vi "Preset_Manager_Main_Integrated.vi"(0 "Cluster":cluster{"Numeric":dbl}, 1 "All Devices Core Info":string[][](array[string]), 2 "Virtual Devices List":string[](array[string]), 3 "Filtered Devices List":string[](array[string]), 4 "DevStatusQueue":refnum<queue>, 5 "UDP timeout ms":i32, 6 "MC Multicast":refnum<k16>, 7 "MCast Remote":u16, 8 "My IP":string, 9 "Experiment Name":string, 10 "Software Root":string, 11 "Mcast address":string) -> ()   [LabVIEW 2020]
uses:
  <vilib>/Utility/miscctls.llb/LVRowAndColumnTypeDef.ctl
  Shared/MySQL/Preset Query Enum.ctl
  <userlib>/_OpenG.lib/array/array.llb/Delete Elements from 1D Array (String)__ogtk.vi
  <userlib>/_OpenG.lib/array/array.llb/openg_array.lvlib
panel:
  in  "EXIT":bool
  in  "Tab Control":T1(tab)
  in  "Execute Preset":bool
  in  "Delete Preset":bool
  in  "Save as Preset":bool
  in  "Preset Menu":u16(ring) items=["None", "Pulsed Alignment", "3J", "Diode", "26J", "SingleShot", "1Hz", "800 MAX ND", "Amp3-8J-CapExit", "SDI", "CapInHexPosition", "CapOutHexFiberPosition", "Full Heater, Frog Out", "Full Heater, Frog In", "MagSpecSimulateBoff", "Pulsed", "CW", "Amp2, Clunker In", "Amp3-17J", "MagSpecSimulateBon", "SMFiber-In", "SMFiber-Out", "Amp3-MegaAttenuator", "developer", "developer_main", "developer_test_1", "dev_simcam_2"]
  in  "View Preset":bool
  in  "Load ECS to Table":bool
  in  "Navigate to ECS File":path
  in  "Preset Table Control":string[][](table)
  in  "Choose Values":bool
  in  "Left Join":bool
  out "Active Preset":string
  in  "Reset Queue":bool
  in  "Queue Table Control":string[][](table)
  in  "Queue Table":string[][](table)
  in  "Execute Queue":bool
  in  "Incoming Preset Refnum":refnum<vi>
  in  "Execute Preset Refnum":refnum<vi>
  out "PRESET FROM DB":string[][](table)
  out "ECS File":string[][](table)
  out "Coordinate Array":i32[][](array[numeric])
  in  "Outgoing Preset Refnum":refnum<vi>
  out "Devices not started":string[](array[string]) caption="Devices not ready for scan"
  out "Active Device array":bool[](array[boolean])
  out "Active Dev/IP":string[](array[string])
  out "Device Errors":string[][](array[string])
  out "error out":errorcluster
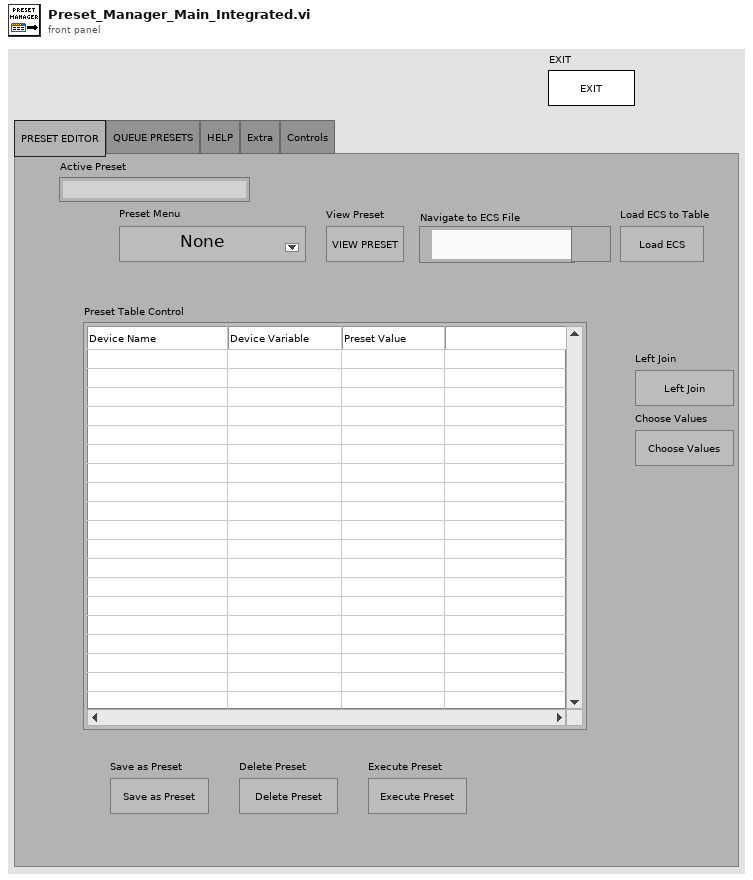
[diagram p1: front panel]
types:
  T1 = enum32{"PRESET EDITOR", "QUEUE PRESETS", "HELP", "Extra", "Controls"}
  T2 = typedef "LVRowAndColumnTypeDef.ctl" = cluster{"Row":i32, "Column":i32}
  T3 = typedef "Preset Query Enum.ctl" = enum16{"Get Locations", "Get all IPs and MACs", "Get classes", "Get expt variables to set at scanstart for particular device", "Get expt devices and variables with start values", "Get expt devices and variables (with data to get)", "Get expt devices with data to get", "Get Expt devices and GUIs", "Get all devices basic properties", "Get Virtual Devices Core Info", "Get Expt names", "Get experiment basic properties", "Get experiment alarm variables", "Get MC Ports", "Get device network comm port", "Get devicetype lvclass path", "Get basic device properties", "Get Init Order", "Get all setable variables of a device", "Get device variable aliases", "Get force values of all settable variables", "Get all variables of a devicetype", "Get all variables of a device", "Get plotter details", "Get Saved Scans", "Get Scan Info", "GetGeneralGUIs", "Get expt for plotter", "Get plotter IDs from expt", "Get all devices", "Get all Virtual Devices", "Get all aliases", "Get variable and device info for Virtual Device", "GetItemLocatorIP", "Get IPs for GUIs", "Get DeviceType from Device", "GetLocalPortRange", "GetDevicePresetVariables", "Get Device Configuration", "GetAllPresetNames", "GetAllConfigurationNames", "GetPresetDeviceNames", "GetDeviceAliases", "GetDevicesOfClass"}
  T4 = enum32{"Invalid", "Standard", "Closed", "Hidden", "Minimized", "Maximized"}
  T5 = enum32{"invalid app kind", "Development System", "Run Time System", "Student Edition", "Embedded LabVIEW", "Evaluation", "Custom"}
  T6 = typedef "LVPoint32TypeDef.ctl" = cluster{"Horizontal":i32, "Vertical":i32}
  T7 = cluster{"Core":cluster{"Current VI Reference":refnum<vi>, "Close Panel on Exit?":bool}, "Your Boolean data":bool, "Your string data":string, "Preset Table Control":string[][], "Column Headers[]":string[], "Temporary Preset":string[][], "Queue Table Control":string[][], "Preset Manager Cluster":cluster{"PresetName":string, "Mcast command":string, "Current Preset Devices":string[], "My IP":string, "Mcast address":string, "Software Root":string, "Experiment Name":string, "MCast Remote":u16, "UDP timeout ms":i32, "MC Multicast":refnum<k16>, "All Devices Core Info":string[][], "Filtered Devices List":string[], "Virtual Devices List":string[], "DevStatusQueue":refnum<queue>}}
  T8 = cluster{"Current VI Reference":refnum<vi>, "Close Panel on Exit?":bool}
  T9 = cluster{"PresetName":string, "Mcast command":string, "Current Preset Devices":string[], "My IP":string, "Mcast address":string, "Software Root":string, "Experiment Name":string, "MCast Remote":u16, "UDP timeout ms":i32, "MC Multicast":refnum<k16>, "All Devices Core Info":string[][], "Filtered Devices List":string[], "Virtual Devices List":string[], "DevStatusQueue":refnum<queue>}
  T10 = enum16{"Left Button", "Center Button", "Right Button", "Window Close"}
  T11 = typedef "mysql_authentication.ctl" = cluster{"User":string, "Password":string, "Database":string}
  T12 = cluster{"Port":u16, "IP Address":string, "Authentication":T11}
  T13 = typedef "preset diagnostics.ctl" = cluster{"Active Preset Achieved":bool, "Devices with Active Preset Not Set":string[], "Dev Presets":string[], "All Preset Devices ON?":bool[]}
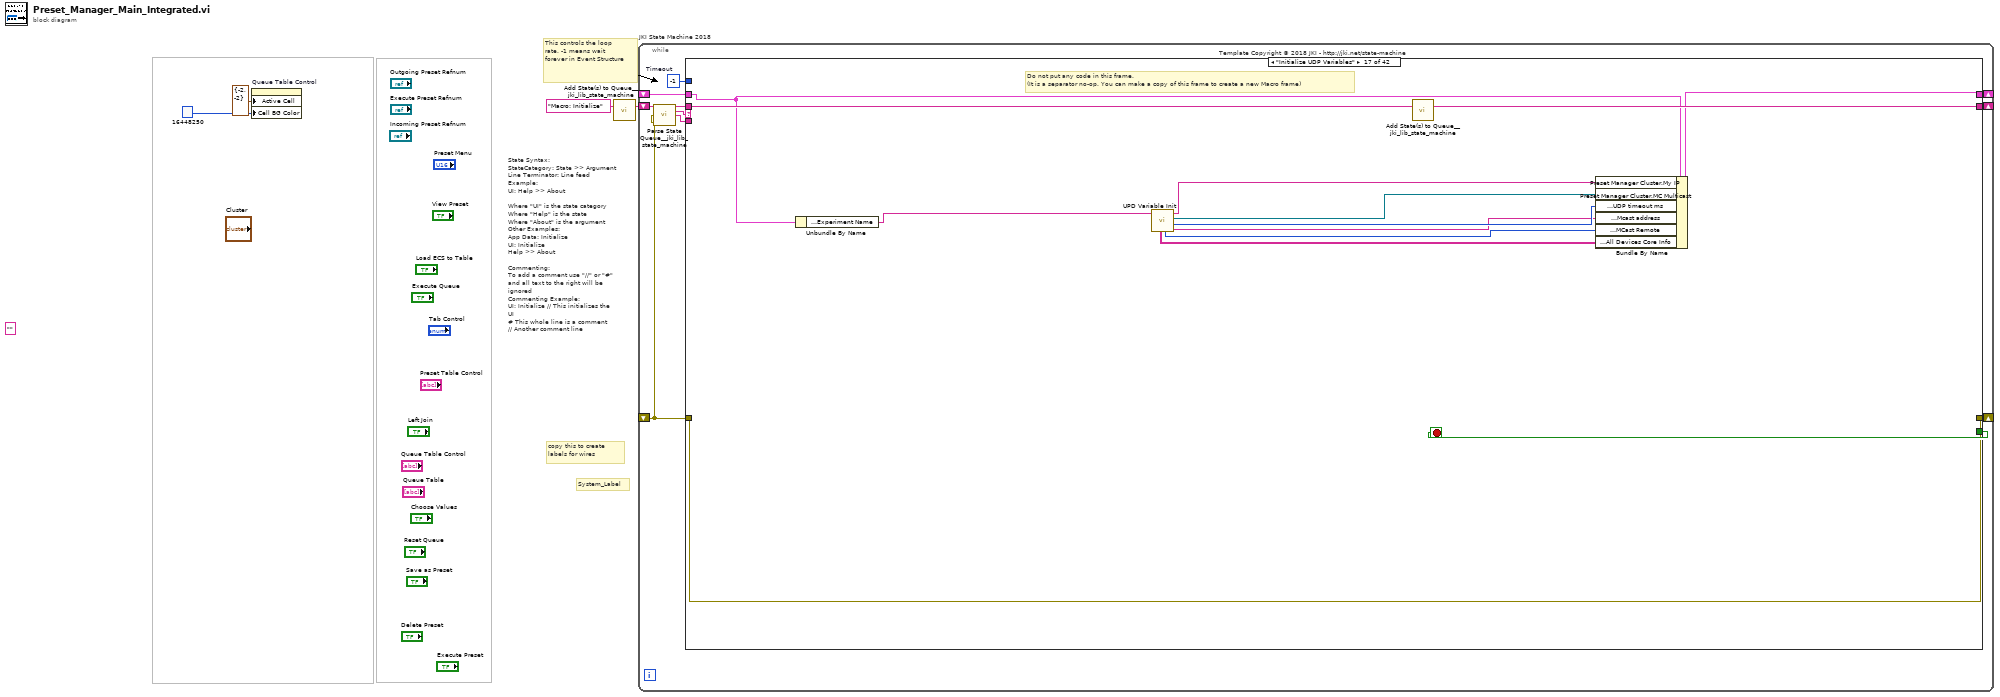
[diagram p0: block diagram]
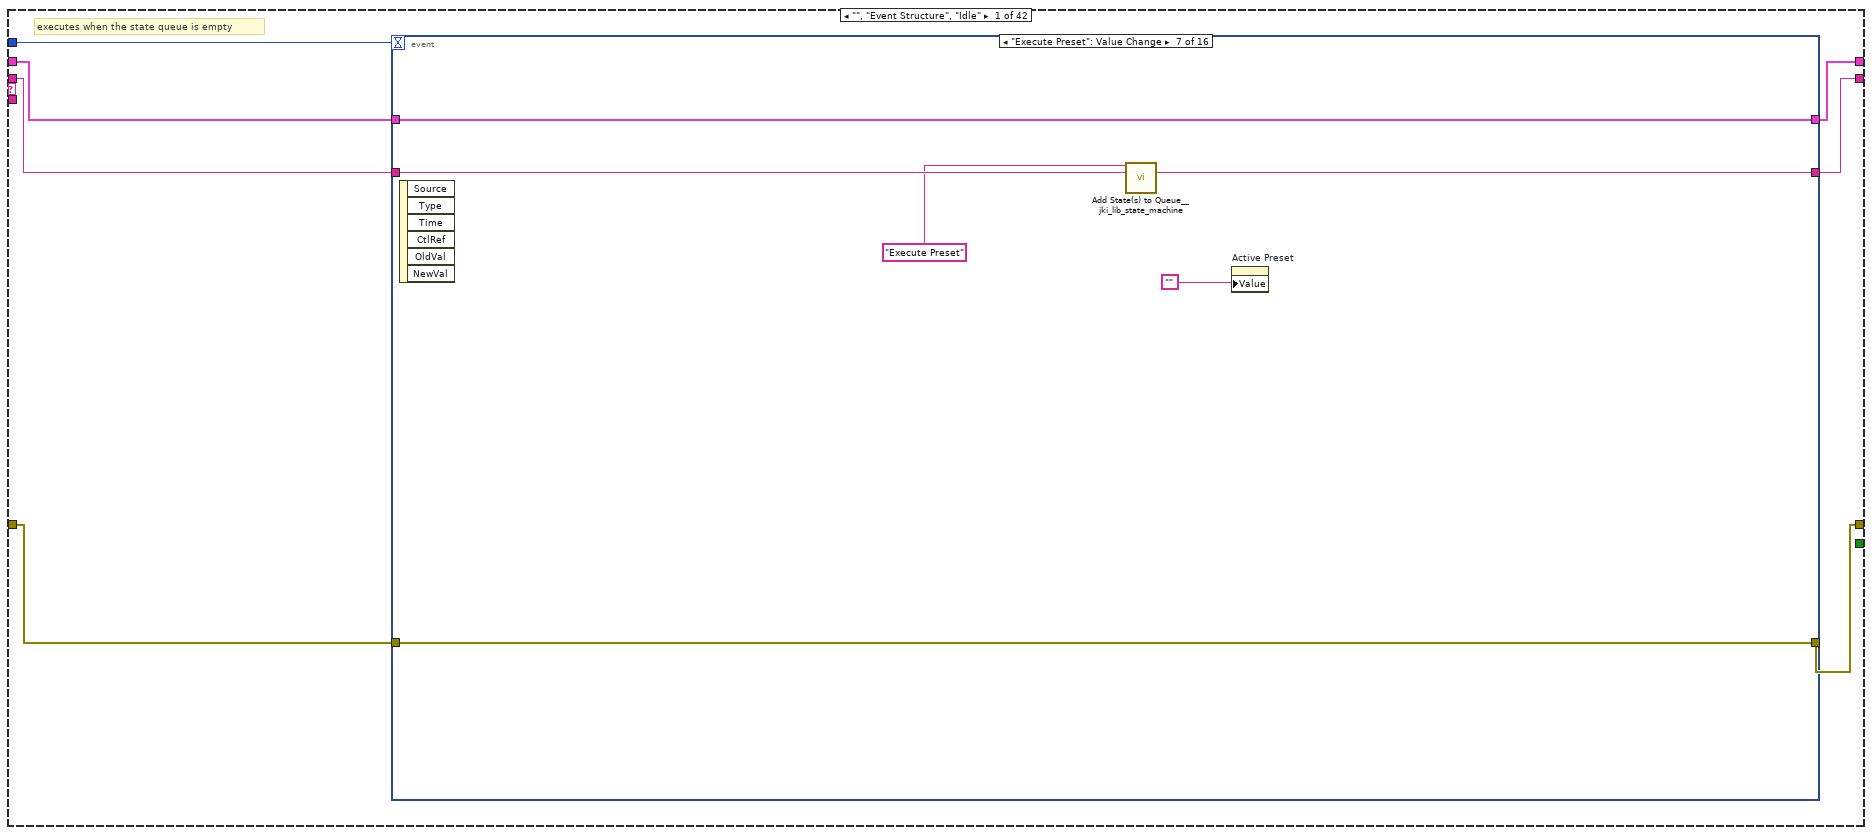
[diagram p2: hidden frame]
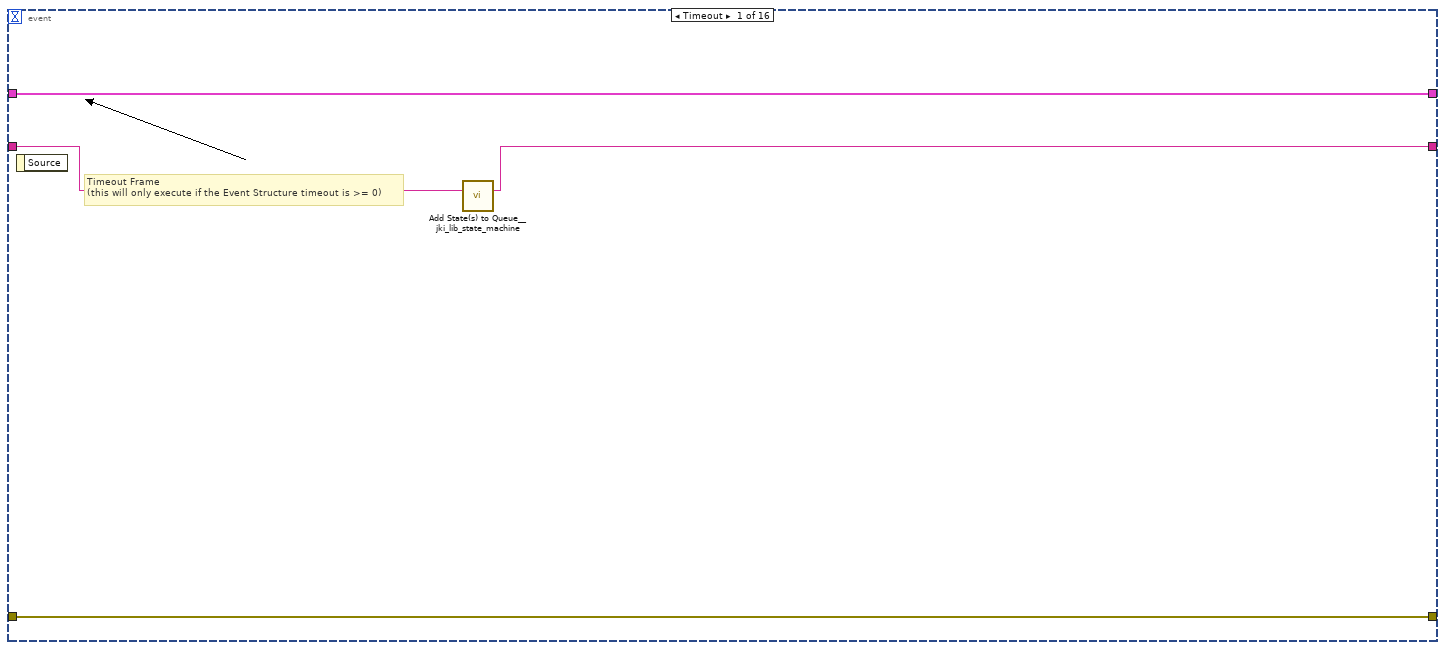
[diagram p3: hidden frame]
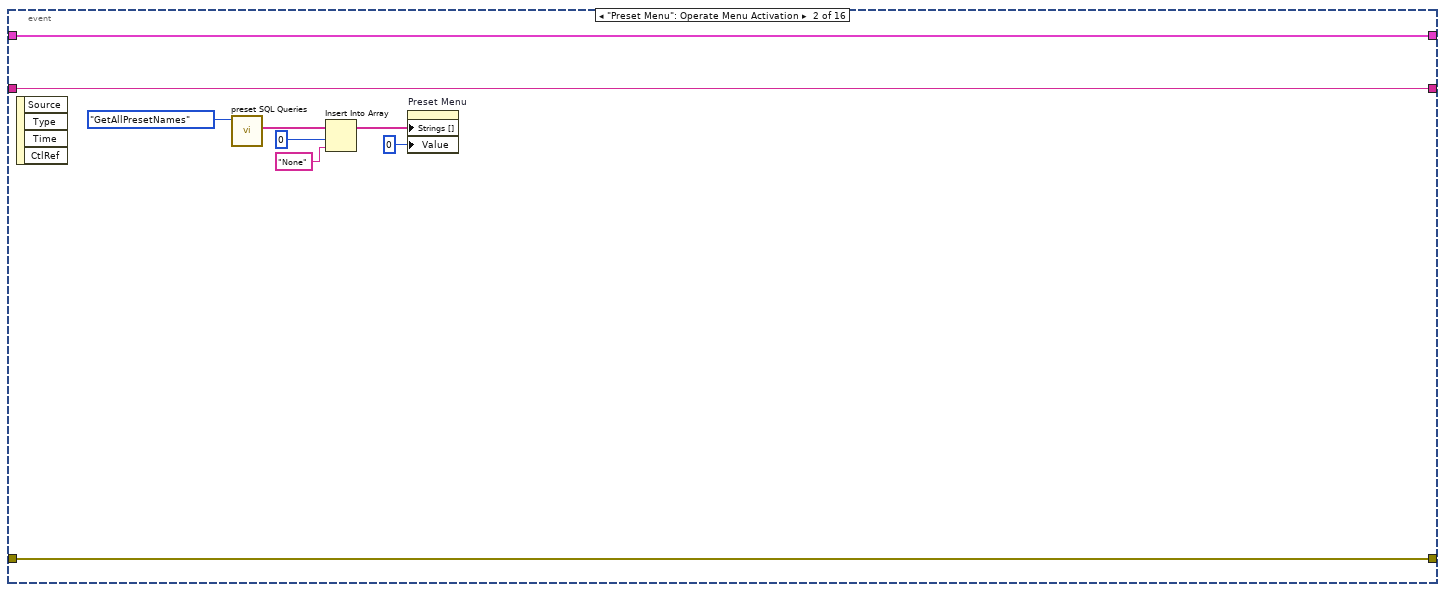
[diagram p4: hidden frame]
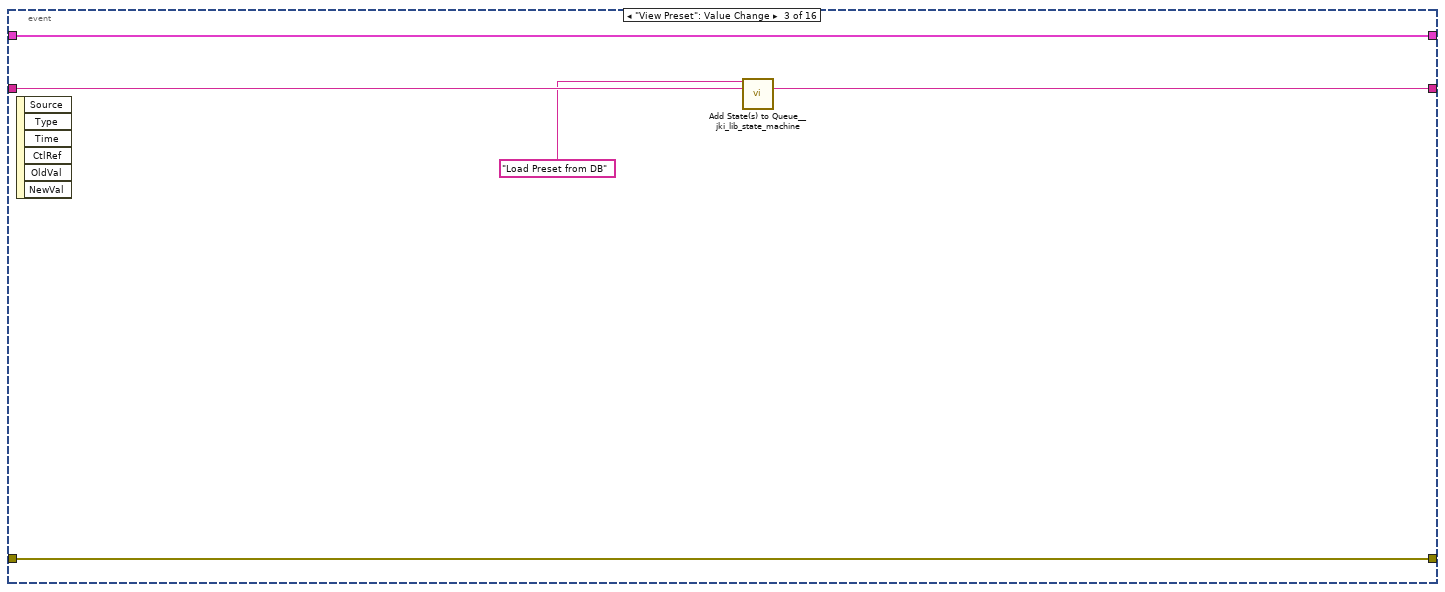
[diagram p5: hidden frame]
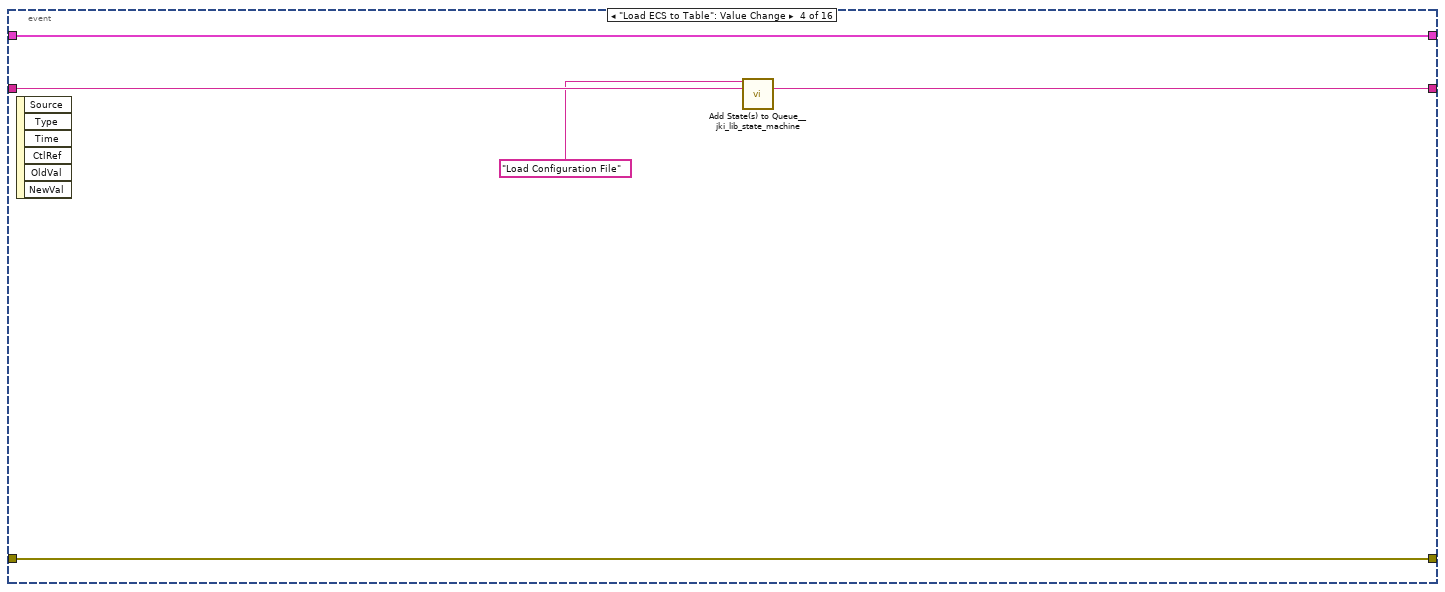
[diagram p6: hidden frame]
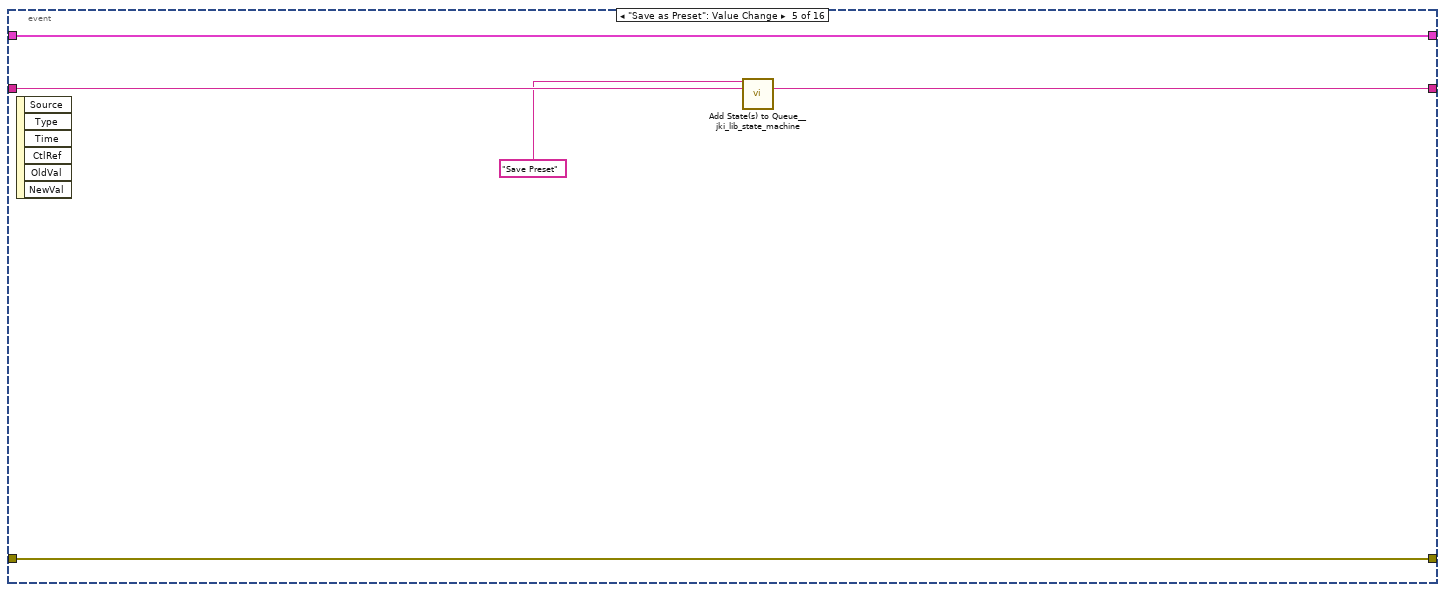
[diagram p7: hidden frame]
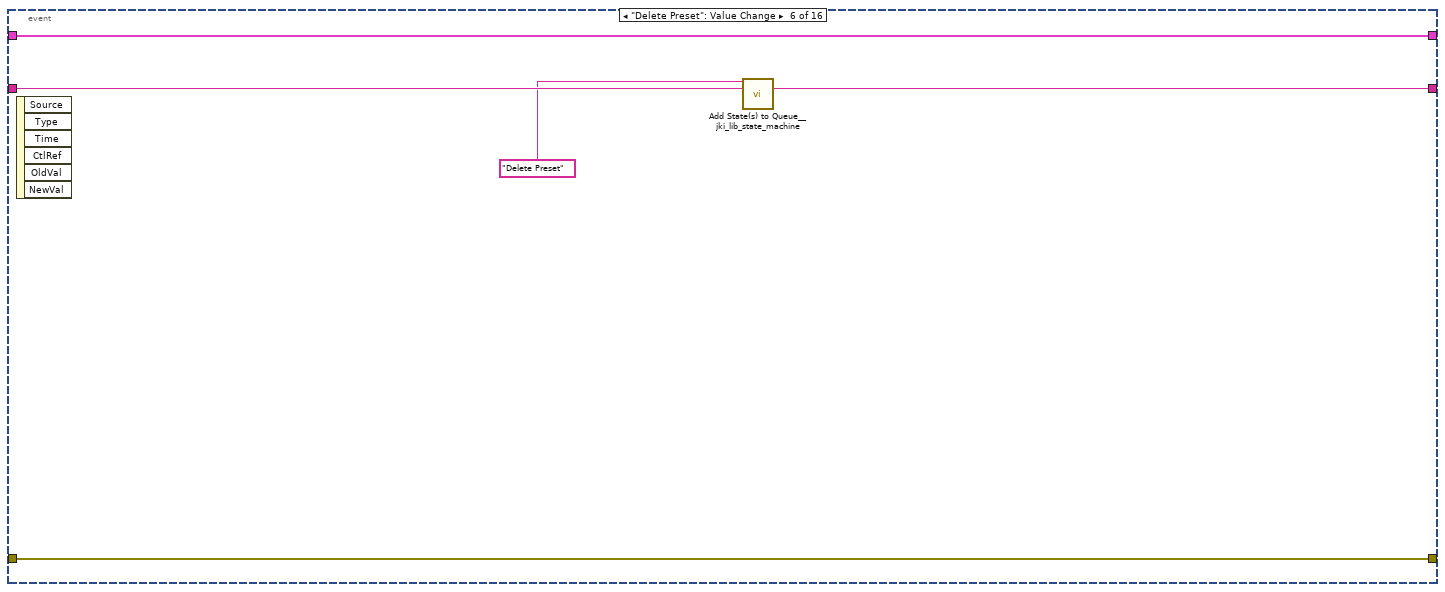
[diagram p8: hidden frame]
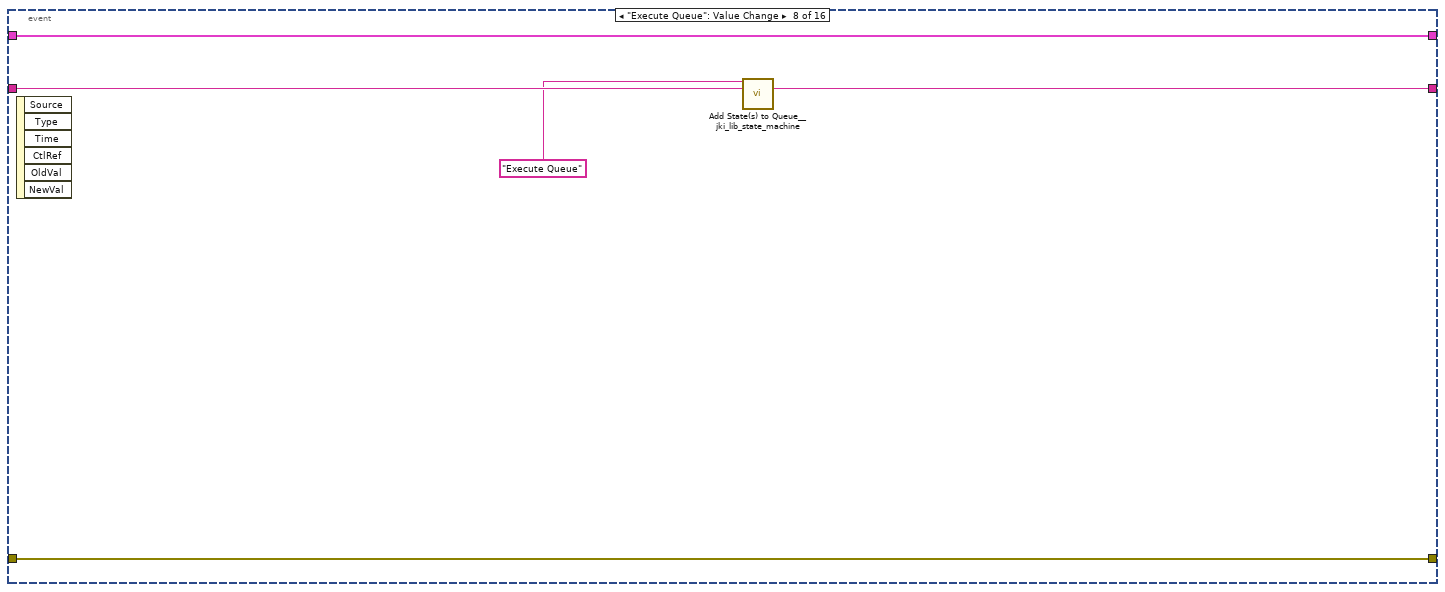
[diagram p9: hidden frame]
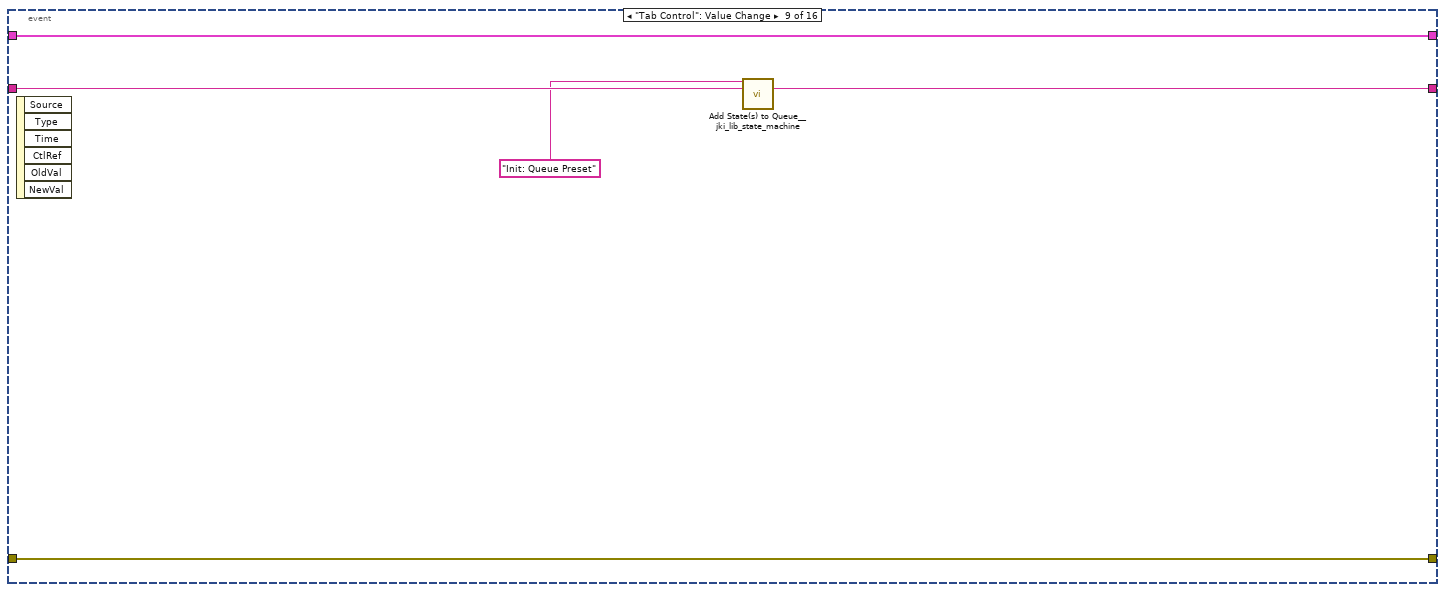
[diagram p10: hidden frame]
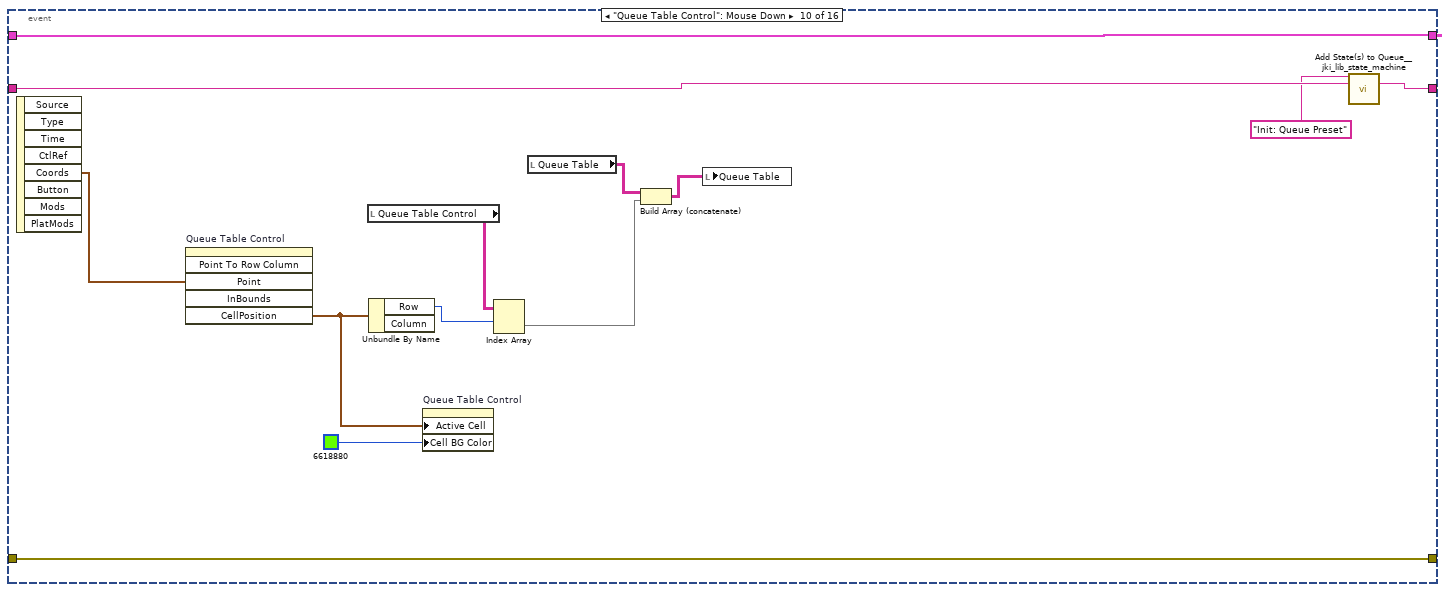
[diagram p11: hidden frame]
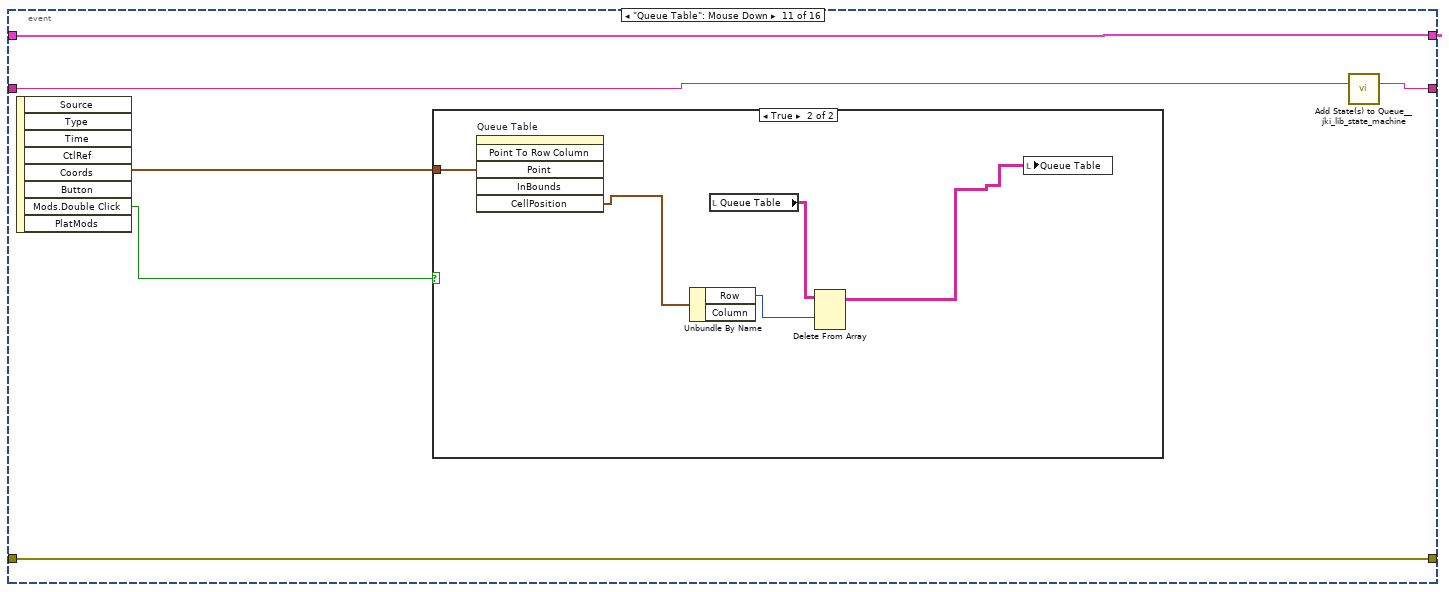
[diagram p12: hidden frame]
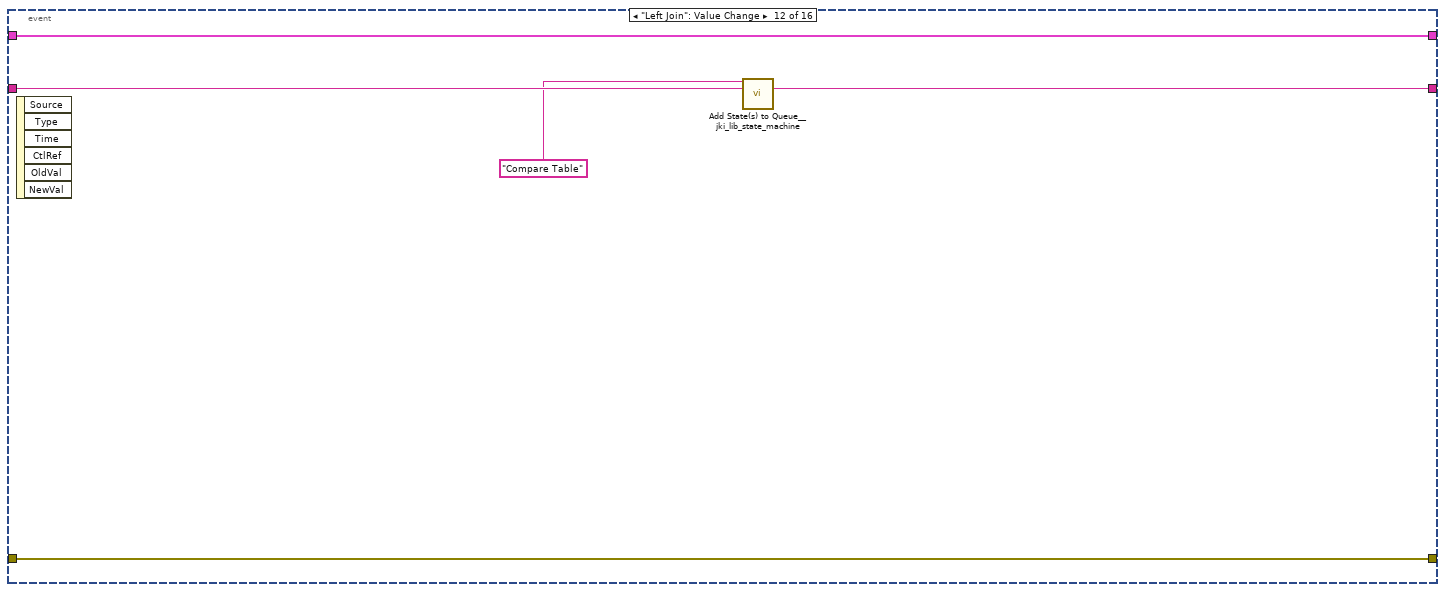
[diagram p14: hidden frame]
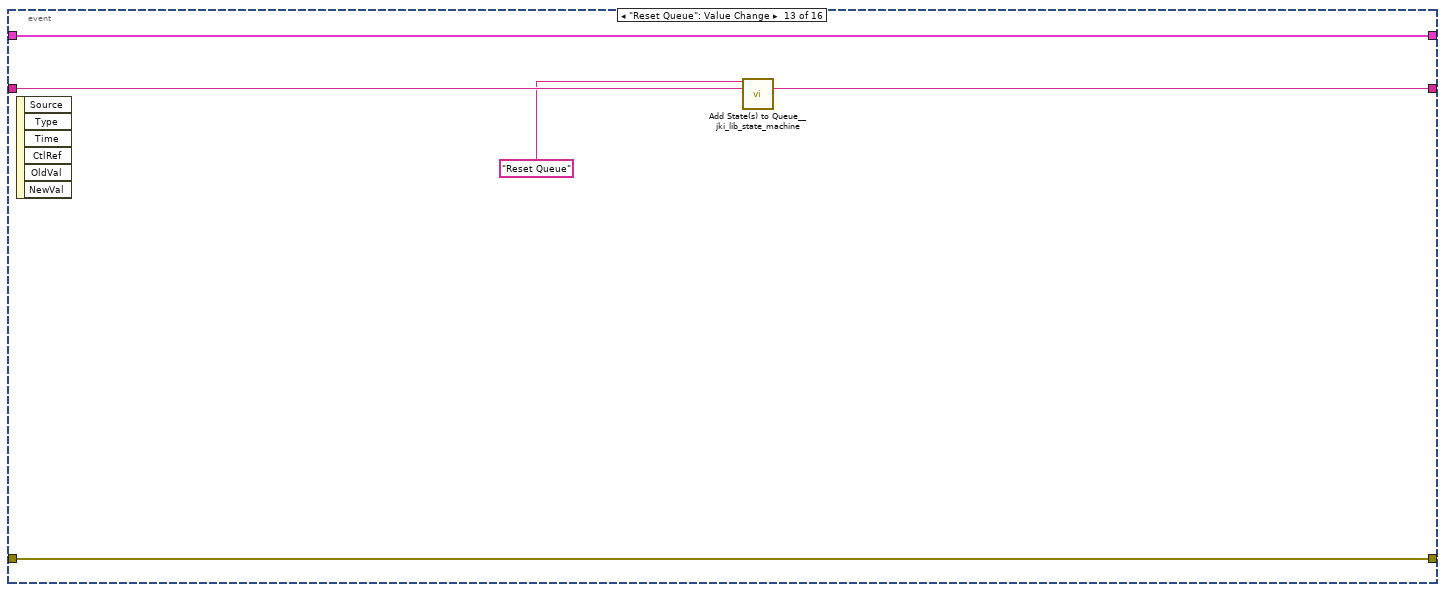
[diagram p15: hidden frame]
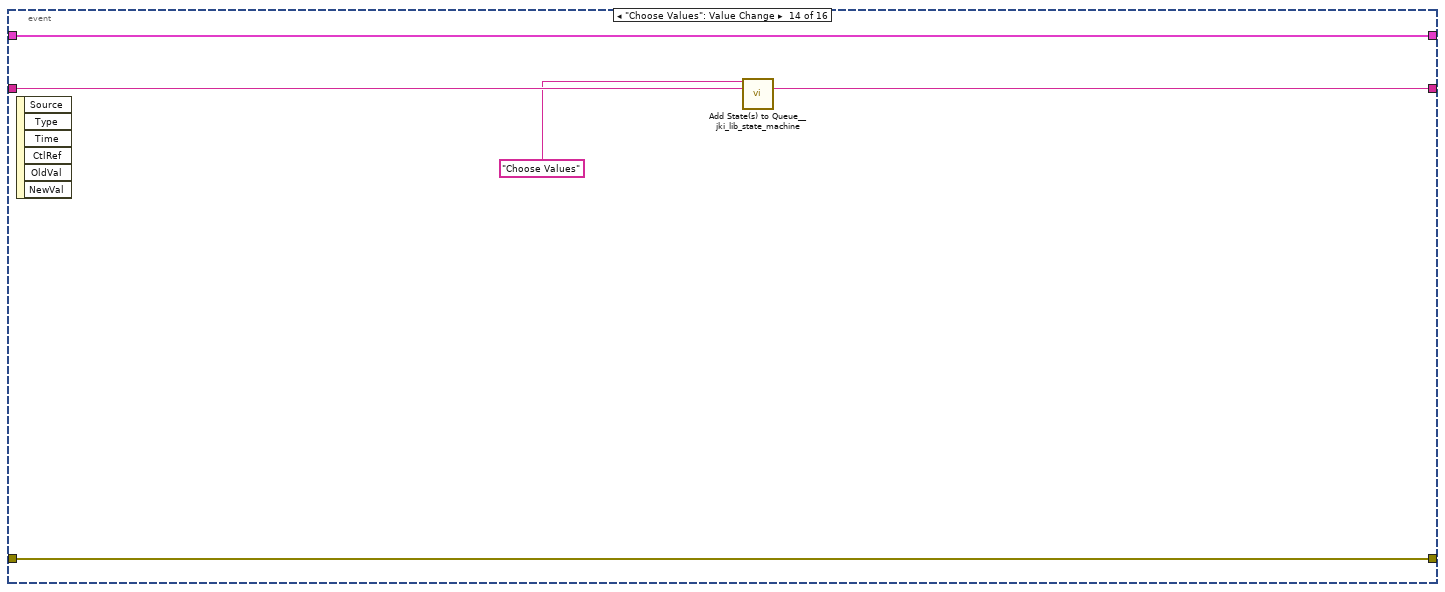
[diagram p16: hidden frame]
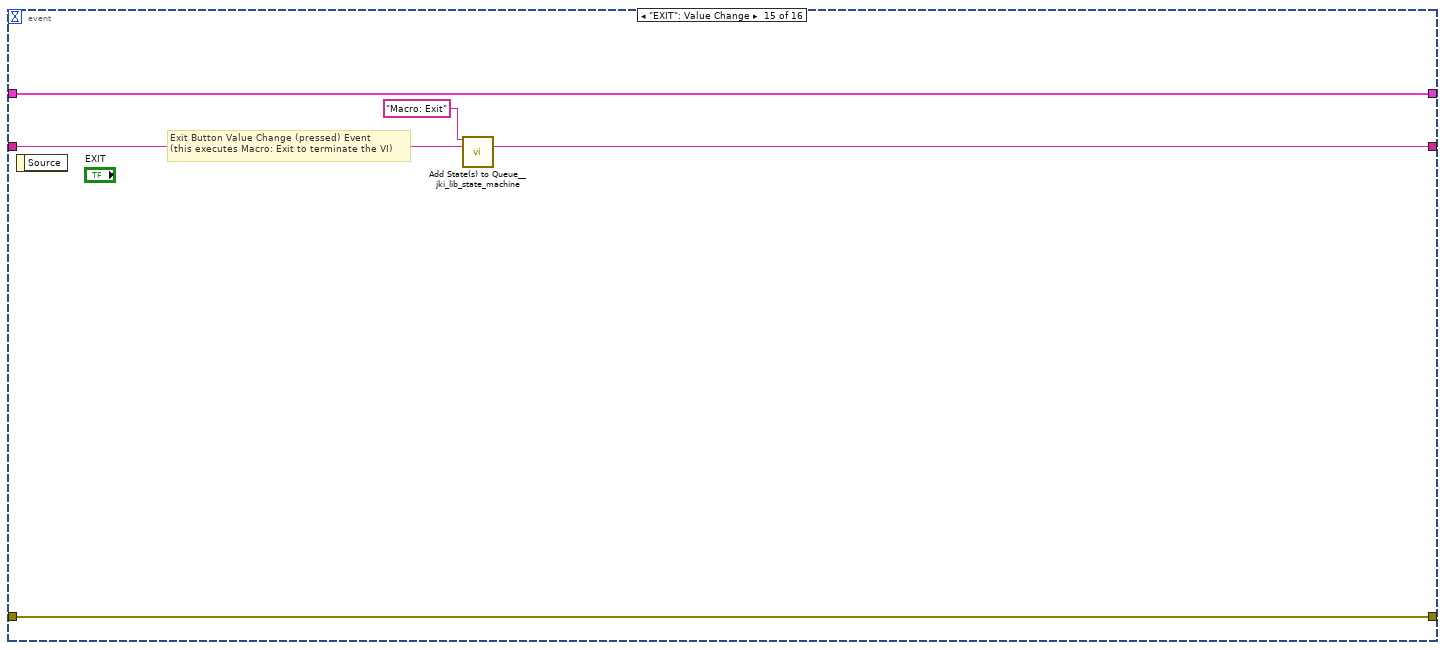
[diagram p17: hidden frame]
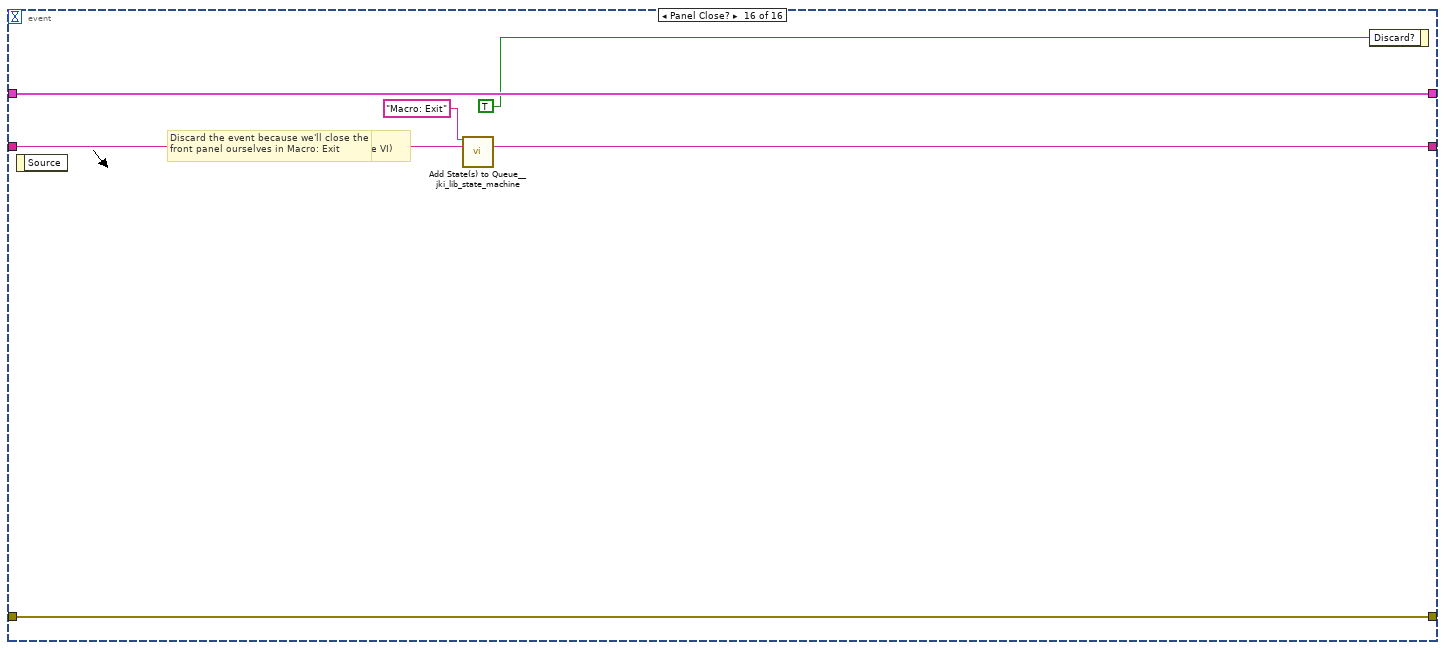
[diagram p18: hidden frame]
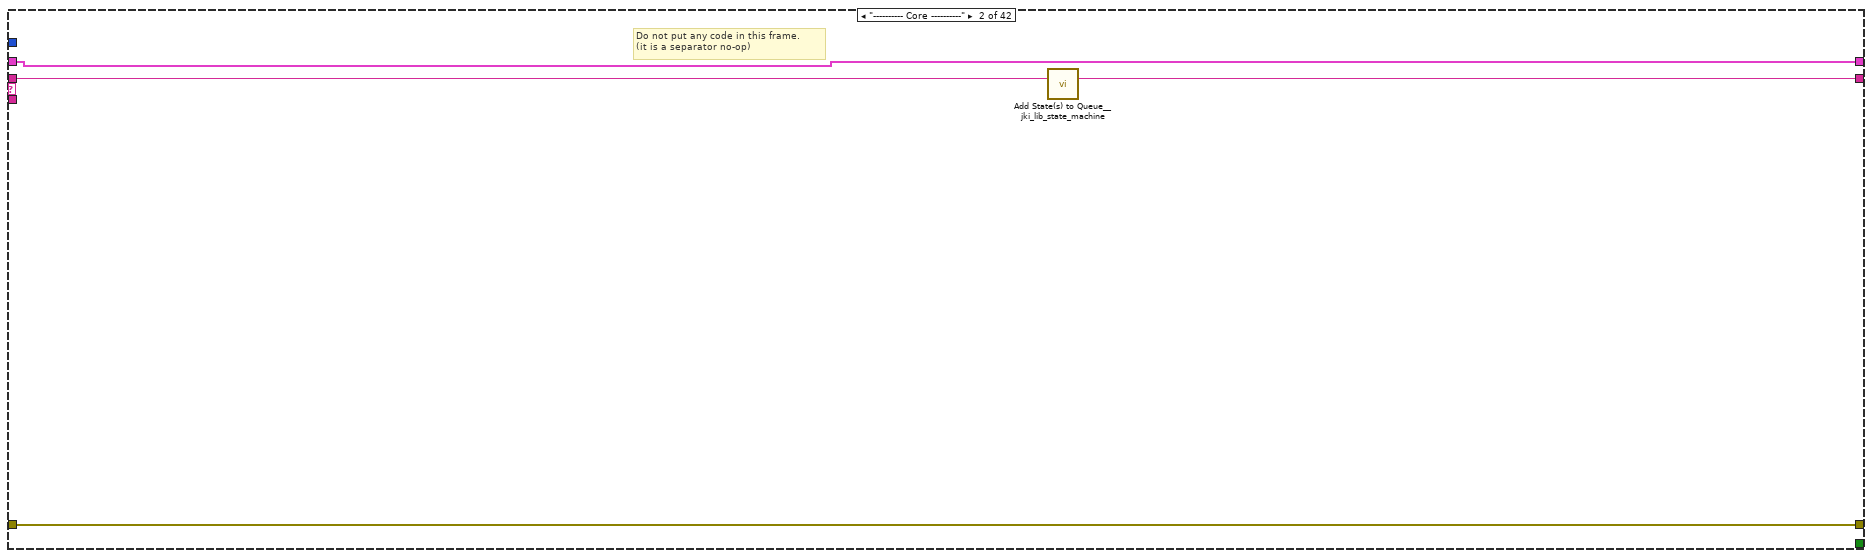
[diagram p19: hidden frame]
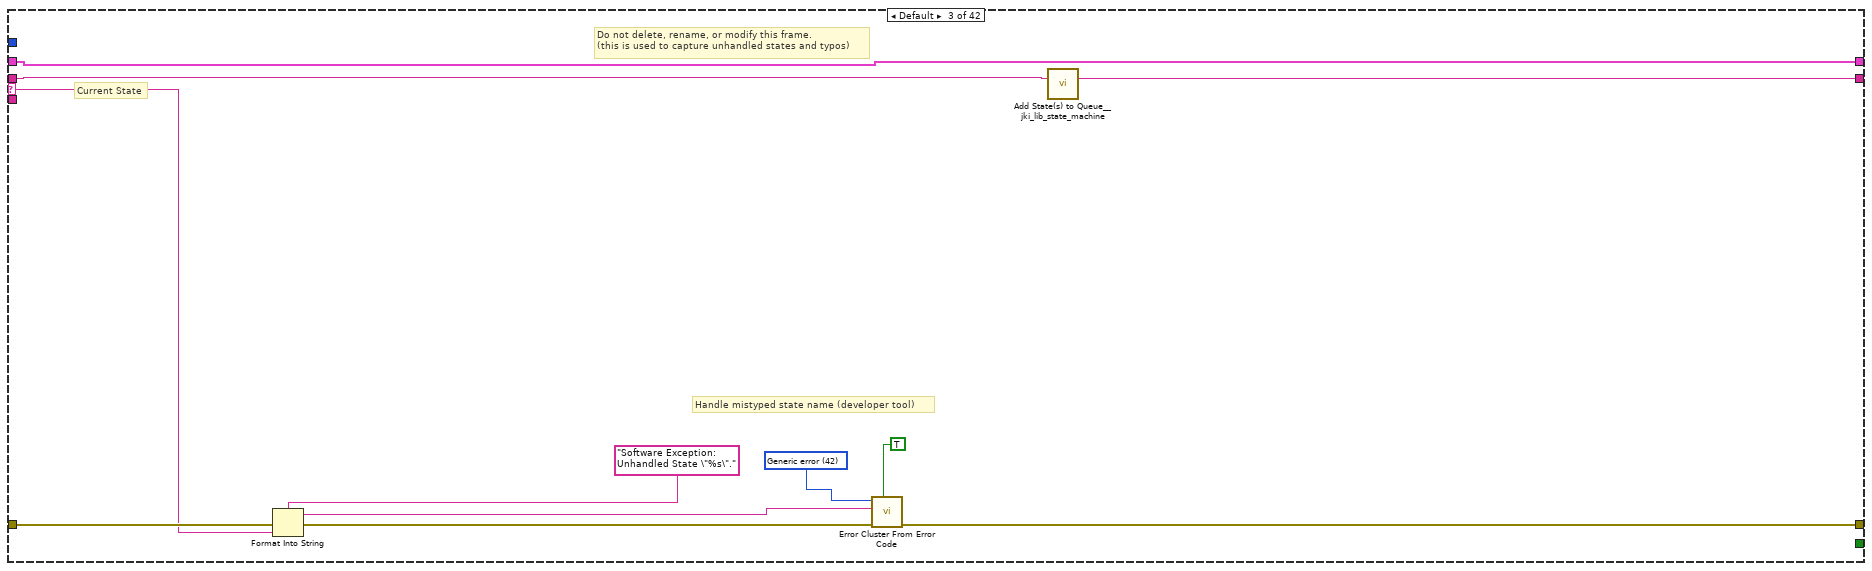
[diagram p20: hidden frame]
diagram:
  (unwired) "" ("My IP")
  # "State Syntax:\nStateCategory: State >> Argument\nLine Terminator: Line feed\nExample:\nUI: Help >> About\n\nWhere \"UI\" is the state category\nWhere \"Help\" is the state\nWhere \"About\" is the argument\nOther Examples:\nApp Data: Initialize\nUI: Initialize\nHelp >> About\n\nCommenting:\nTo add a comment use \"//\" or \"#\" and all text to the right will be ignored\nCommenting Example:\nUI: Initialize // This initializes the UI\n# This whole line is a comment\n// Another comment line"
  # "copy this to create labels for wires"
  # "This controls the loop rate. -1 means wait forever in Event Structure"
  # "System_Label"
  n1 = property on="Queue Table Control" class="Tbl (strict)"("Active Cell"=T2 {"Row"=-2, "Column"=-2} ("Active Cell:Active Cell"), "Cell BG Color"=u32 16448250 ("Active Cell:Cell Background Color")) -> ()  [unwired: 2 in, 2 out]
  n2 = call <vilib>:"Add State(s) to Queue__jki_lib_state_machine.vi"("State(s) in (\"\")"="Macro: Initialize") -> ("States Out"=w4:string)  [unwired: 14 in]
  n3 = while "JKI State Machine 2018" {
    shift-right: [w5] -> _
    shift-left: _ -> [w8]
    shift-right: [w11] -> _
    shift-left: _ -> [w6]
    shift-right: [w10] -> _
    shift-left: w4 -> [w12]
    stop <- w9 stop-if-true
    w7 = -1  # Timeout
    # "Template Copyright © 2018 JKI - http://jki.net/state-machine"
    n4 = call <vilib>:"Parse State Queue__jki_lib_state_machine.vi"("State Queue"=w12, "Error In (no error)"=w6) -> ("Remaining States"=w14:string, "Current State"=w15:string, "Arguments"=w13:string)  [unwired: 11 in]
    n5 = case shown="\"Initialize UDP Variables\"" w15 {
      selector: w15 -> [_ _ w126 _ _ _ _ _ _ _ _ _ _ _ _ _ _ _ _ _ _ _ _ _ _ _ _ _ _ _ _ _ _ _ _ _ _ _ _ _ _ _]
      tunnel: w14 -> [w22 w125 w130 w149 w155 w160 w164 w182 w188 w192 w196 w202 w213 w282 w287 w297 w309 w313 w323 w331 w341 w350 w359 w369 w386 w412 w446 w458 w462 w466 w470 w476 w480 w487 w496 w505 w527 w538 w545 w563 w589 w601]
      tunnel: w13 -> [_ _ _ _ _ _ _ _ _ _ _ w197 w207 _ _ _ _ _ _ _ _ _ _ _ _ _ _ _ _ _ _ _ _ _ _ _ _ _ w539 _ _ _]
      tunnel: w8 -> [w20 w122 w128 w142 w152 w158 w161 _ w183 w189 w194 w200 w209 w279 w284 w294 w306 w310 w318 w324 w337 w347 w355 w366 w383 w409 w442 w455 w459 w463 w467 w473 w477 w482 w493 w501 w524 w535 w542 w559 w581 w592]
      tunnel: [w19 w123 w132 w146 errorcluster {"status"=FALSE, "code"=0, "source"=""} ("error out") w157 w162 w180 w184 w190 w193 w198 w210 w280 w285 w295 w307 w311 w321 w329 w339 w348 w357 w367 w384 w410 w444 w456 w460 w464 w468 w474 w478 w485 w494 w503 w525 w536 w543 w561 w587 w599] -> w11
      tunnel: w6 -> [w18 w123 w131 w146 w151 w157 w162 w180 w185 w190 w193 w199 w211 w280 w285 w295 w307 w311 w321 w329 w339 w348 w357 w367 w384 w410 w444 w456 w460 w464 w468 w474 w478 w485 w494 w503 w525 w536 w543 w561 w587 w599]
      tunnel: [w21 w124 w129 w148 w154 w159 w163 w181 w187 w191 w195 w201 w212 w281 w286 w296 w308 w312 w322 w330 w340 w349 w358 w368 w385 w411 w445 w457 w461 w465 w469 w475 w479 w486 w495 w504 w526 w537 w544 w562 w588 w600] -> w10
      tunnel: [_ _ _ _ _ TRUE _ _ _ _ _ _ _ _ _ _ _ _ _ _ _ _ _ _ _ _ _ _ _ _ _ _ _ _ _ _ _ _ _ _ _ _] -> w9
      tunnel: w7 -> [w16 _ _ _ _ _ _ _ _ _ _ _ _ _ _ _ _ _ _ _ _ _ _ _ _ _ _ _ _ _ _ _ _ _ _ _ _ _ _ _ _ _]
      tunnel: [w17 w122 w128 w147 w152 w158 w161 w170 w183 w189 w194 w200 w209 w279 w284 w294 w305 w310 w316 w324 w336 w346 w354 w366 w383 w409 w442 w455 w459 w463 w467 w473 w477 w482 w493 w501 w524 w528 w542 w559 w582 w590] -> w5
      frame "", "Event Structure", "Idle" {
        # "executes when the state queue is empty"
        n6 = event shown="[6] \"Execute Preset\": Value Change" {
          selector: _ -> [_ _ _ _ _ _ _ _ _ _ _ _ _ _ _ _]
          dyn-events: _ -> [_ _ _ _ _ _ _ _ _ _ _ _ _ _ _ _]
          timeout: w16 -> [_ _ _ _ _ _ _ _ _ _ _ _ _ _ _ _]
          tunnel: w22 -> [w26 w34 w38 w43 w48 w53 w59 w64 w70 w83 w89 w98 w103 w108 w115 w121]
          tunnel: [w25 w34 w37 w42 w47 w52 w58 w63 w69 w82 w88 w97 w102 w107 w114 w120] -> w21
          tunnel: w20 -> [w23 w35 w40 w45 w50 w55 w61 w66 w67 w80 w87 w100 w105 w110 w112 w118]
          tunnel: [w24 w33 w39 w44 w49 w54 w60 w65 w71 w84 w90 w99 w104 w109 w113 w119] -> w19
          tunnel: w18 -> [w24 w33 w39 w44 w49 w54 w60 w65 w71 w84 w90 w99 w104 w109 w113 w119]
          tunnel: [w23 w35 w40 w45 w50 w55 w61 w66 w67 w80 w87 w100 w105 w110 w112 w118] -> w17
          event Timeout {
            # "Timeout Frame\n(this will only execute if the Event Structure timeout is >= 0)"
            n7 = event-data() -> ()  [unwired: 1 in, 1 out]
            n8 = call <vilib>:"Add State(s) to Queue__jki_lib_state_machine.vi"("State(s) in (\"\")"=w26) -> ("States Out"=w25:string)  [unwired: 14 in]
          }
          event "Preset Menu": Operate Menu Activation {
            n9 = event-data() -> ()  [unwired: 1 in, 4 out]
            n10 = call "preset SQL Queries.vi"("Preset Query"=Preset_Query_Enum."GetAllPresetNames") -> ("1st column 1st data"=w31:string[])  [unwired: 8 in, 2 out]
            n11 = Insert Into Array(array=w31, index=0, new element="None" ("new element/subarray")) -> (w28:string[])
            n12 = property on="Preset Menu" class="Ring (strict)"("Strings []"=w28, "Value"=0 ("index")) -> ()  [unwired: 2 in, 2 out]
          }
          event "View Preset": Value Change {
            n13 = event-data() -> ()  [unwired: 1 in, 6 out]
            n14 = call <vilib>:"Add State(s) to Queue__jki_lib_state_machine.vi"("State(s) in Front (\"\")"="Load Preset from DB", "State(s) in (\"\")"=w38) -> ("States Out"=w37:string)  [unwired: 13 in]
          }
          event "Load ECS to Table": Value Change {
            n15 = event-data() -> ()  [unwired: 1 in, 6 out]
            n16 = call <vilib>:"Add State(s) to Queue__jki_lib_state_machine.vi"("State(s) in Front (\"\")"="Load Configuration File", "State(s) in (\"\")"=w43) -> ("States Out"=w42:string)  [unwired: 13 in]
          }
          event "Save as Preset": Value Change {
            n17 = event-data() -> ()  [unwired: 1 in, 6 out]
            n18 = call <vilib>:"Add State(s) to Queue__jki_lib_state_machine.vi"("State(s) in Front (\"\")"="Save Preset", "State(s) in (\"\")"=w48) -> ("States Out"=w47:string)  [unwired: 13 in]
          }
          event "Delete Preset": Value Change {
            n19 = event-data() -> ()  [unwired: 1 in, 6 out]
            n20 = call <vilib>:"Add State(s) to Queue__jki_lib_state_machine.vi"("State(s) in Front (\"\")"="Delete Preset", "State(s) in (\"\")"=w53) -> ("States Out"=w52:string)  [unwired: 13 in]
          }
          event "Execute Preset": Value Change {
            n21 = event-data() -> ()  [unwired: 1 in, 6 out]
            n22 = call <vilib>:"Add State(s) to Queue__jki_lib_state_machine.vi"("State(s) in Front (\"\")"="Execute Preset", "State(s) in (\"\")"=w59) -> ("States Out"=w58:string)  [unwired: 13 in]
            n23 = property on="Active Preset" class="Str"("Value"="") -> ()  [unwired: 2 in, 2 out]
          }
          event "Execute Queue": Value Change {
            n24 = event-data() -> ()  [unwired: 1 in, 6 out]
            n25 = call <vilib>:"Add State(s) to Queue__jki_lib_state_machine.vi"("State(s) in Front (\"\")"="Execute Queue", "State(s) in (\"\")"=w64) -> ("States Out"=w63:string)  [unwired: 13 in]
          }
          event "Tab Control": Value Change {
            n26 = event-data() -> ()  [unwired: 1 in, 6 out]
            n27 = call <vilib>:"Add State(s) to Queue__jki_lib_state_machine.vi"("State(s) in Front (\"\")"="Init: Queue Preset", "State(s) in (\"\")"=w70) -> ("States Out"=w69:string)  [unwired: 13 in]
          }
          event "Queue Table Control": Mouse Down {
            n28 = event-data() -> ("Coords"=w79:T6)  [unwired: 1 in, 7 out]
            n29 = invoke on="Queue Table Control" class="Tbl (strict)" method="Point To Row Column"("Point"=w79) -> ("CellPosition"=w76:T2)  [unwired: 5 in, 5 out]
            n30 = local read "Queue Table Control"() -> (w78:string[][])
            n31 = Unbundle By Name(w76) -> ("Row"=w77:i32)  [unwired: 1 out]
            n32 = property on="Queue Table Control" class="Tbl (strict)"("Active Cell"=w76, "Cell BG Color"=u32 6618880 ("Active Cell:Cell Background Color")) -> ()  [unwired: 2 in, 2 out]
            n33 = Index Array(array=w78, index (row)=w77) -> (element=w74:string[])  [unwired: 1 in]
            n34 = local read "Queue Table"() -> (w72:string[][])
            n35 = Build Array (concatenate)(w72, w74) -> (w73:string[][])
            n36 = local write "Queue Table"(w73) -> ()
            n37 = call <vilib>:"Add State(s) to Queue__jki_lib_state_machine.vi"("State(s) in Front (\"\")"="Init: Queue Preset", "State(s) in (\"\")"=w83) -> ("States Out"=w82:string)  [unwired: 13 in]
          }
          event "Queue Table": Mouse Down {
            n38 = event-data() -> ("Coords"=w86:T6, "Mods.Double Click"=w85:bool)  [unwired: 1 in, 6 out]
            n39 = case shown="True" w85 {
              tunnel: w86 -> [_ w94]
              frame False {
              }
              frame True {
                n40 = invoke on="Queue Table" class="Tbl (strict)" method="Point To Row Column"("Point"=w94) -> ("CellPosition"=w93:T2)  [unwired: 5 in, 5 out]
                n41 = Unbundle By Name(w93) -> ("Row"=w91:i32)  [unwired: 1 out]
                n42 = local read "Queue Table"() -> (w95:string[][])
                n43 = Delete From Array(array=w95, index (row)=w91) -> (array with subset deleted=w92:string[][])  [unwired: 2 in, 1 out]
                n44 = local write "Queue Table"(w92) -> ()
              }
            }
            n45 = call <vilib>:"Add State(s) to Queue__jki_lib_state_machine.vi"("State(s) in (\"\")"=w89) -> ("States Out"=w88:string)  [unwired: 14 in]
          }
          event "Left Join": Value Change {
            n46 = event-data() -> ()  [unwired: 1 in, 6 out]
            n47 = call <vilib>:"Add State(s) to Queue__jki_lib_state_machine.vi"("State(s) in Front (\"\")"="Compare Table", "State(s) in (\"\")"=w98) -> ("States Out"=w97:string)  [unwired: 13 in]
          }
          event "Reset Queue": Value Change {
            n48 = event-data() -> ()  [unwired: 1 in, 6 out]
            n49 = call <vilib>:"Add State(s) to Queue__jki_lib_state_machine.vi"("State(s) in Front (\"\")"="Reset Queue", "State(s) in (\"\")"=w103) -> ("States Out"=w102:string)  [unwired: 13 in]
          }
          event "Choose Values": Value Change {
            n50 = event-data() -> ()  [unwired: 1 in, 6 out]
            n51 = call <vilib>:"Add State(s) to Queue__jki_lib_state_machine.vi"("State(s) in Front (\"\")"="Choose Values", "State(s) in (\"\")"=w108) -> ("States Out"=w107:string)  [unwired: 13 in]
          }
          event "EXIT": Value Change {
            # "Exit Button Value Change (pressed) Event\n(this executes Macro: Exit to terminate the VI)"
            n52 = event-data() -> ()  [unwired: 1 in, 1 out]
            n53 = call <vilib>:"Add State(s) to Queue__jki_lib_state_machine.vi"("State(s) in Front (\"\")"="Macro: Exit", "State(s) in (\"\")"=w115) -> ("States Out"=w114:string)  [unwired: 13 in]
          }
          event Panel Close? {
            # "Discard the event because we'll close the front panel ourselves in Macro: Exit"
            # "Close Panel button (pressed) Event\n(this executes Macro: Exit to terminate the VI)"
            n54 = event-data() -> ()  [unwired: 1 in, 1 out]
            n55 = call <vilib>:"Add State(s) to Queue__jki_lib_state_machine.vi"("State(s) in Front (\"\")"="Macro: Exit", "State(s) in (\"\")"=w121) -> ("States Out"=w120:string)  [unwired: 13 in]
            n56 = event-data("Discard?"=TRUE) -> ()  [unwired: 1 in, 1 out]
          }
        }
      }
      frame "---------- Core ----------" {
        # "Do not put any code in this frame.\n(it is a separator no-op)"
        n57 = call <vilib>:"Add State(s) to Queue__jki_lib_state_machine.vi"("State(s) in (\"\")"=w125) -> ("States Out"=w124:string)  [unwired: 14 in]
      }
      frame Default {
        w135 = 42 items=["No error", "Argument error", "Memory is full", "Out of zone", "End of file", "File already open", "Generic file I/O error", "File not found", "File permission error", "Disk is full", "Duplicate path", "Too many files open", "System feature not enabled", "Resource file not found", "Cannot add resource", "Resource not found", "Image not found", "Image memory error", "Pen does not exist", "Config type invalid", "Config token not found", "Config parse error", "Config memory error", "Bad external code format", "Bad external code offset", "External code not present", "Null window", "Destroy window error", "Null menu", "Print aborted", "Bad print record", "Print driver error", "Windows error during printing", "Memory error during printing", "Print dialog error", "Generic print error", "Invalid device refnum", "Device not found", "Device parameter error", "Device unit error", "Cannot open device", "Device call aborted", "Generic error", "Cancelled by user", "Object ID too low", "Object ID too high", "Object not in heap", "Unknown heap", "Unknown object (invalid DefProc)", "Unknown object (DefProc not in table)", "Message out of range", "Invalid (null) method", "Unknown message", "Manager call not supported", "Bad address", "Network operation in progress", "Network operation timed out", "Connection is busy", "Network attribute not supported", "Network error", "Address in use", "System out of memory", "Connection aborted", "Connection refused", "Not connected", "Already connected", "Connection closed", "Initialization error (interapplication manager)", "Bad occurrence", "Wait on unbound occurrence handler", "Occurrence queue overflow", "Datalog type conflict", "Unused", "Unrecognized type (interapplication manager)", "Memory corrupt", "Failed to make temporary DLL", "Old CIN version", "Drag socket not found", "Failed to load drop-object", "Failed to register OLE object", "Failed to release OLE object", "Format specifier type mismatch", "Unknown format specifier", "Too few format specifiers", "Too many format specifiers", "Scan failed", "Newer CIN version", "Error converting to variant", "Runtime menu error", "Password tampered", "Variant attribute not found", "Incompatible variant data type", "Event data is not available", "Event Store is not present", "Occurrence is not found", "Event Queue is not created", "Event info is not available", "Refnum passed is NULL", "Error retrieving Class GUID", "Error retrieving CoClass GUID", "Error retrieving TypeLib GUID.", "Bad built application magic bytes.", "Specific driver is different from the specific driver associated with the Logical Name.", "There is no session opened to the class driver.", "Max Error", "MAX - Error with config objects", "MAX - Error loading configuration", "MAX - Group not supported"]
        # "Current State"
        # "Do not delete, rename, or modify this frame.\n(this is used to capture unhandled states and typos)"
        # "Handle mistyped state name (developer tool)"
        n58 = Format Into String(format string="Software Exception: Unhandled State \"%s\"." ("message"), error in=w131, w126) -> (resulting string=w134:string, error out=w133:errorcluster)  [unwired: 1 in]
        n59 = call <vilib>:"Error Cluster From Error Code.vi"("show call chain? (False)"=TRUE, "error in (no error)"=w133, "error message (\"\")"=w134, "error code (0)"=w135) -> ("error out"=w132:errorcluster)  [unwired: 5 in]
        n60 = call <vilib>:"Add State(s) to Queue__jki_lib_state_machine.vi"("State(s) in (\"\")"=w130) -> ("States Out"=w129:string)  [unwired: 14 in]
      }
      frame "Initialize Core Data" {
        # "Do not delete, rename, or modify this frame.\n(this is used to determine panel behavior on exit)"
        # "originally closed?"
        # "exe?"
        # "If panel starts closed or is an EXE, then close it when we exit"
        n61 = property class="VI"() -> ("FP.State"=w139:T4)  [unwired: 2 in, 2 out]
        n62 = property class="App"() -> ("App.Kind"=w145:T5)  [unwired: 2 in, 2 out]
        n63 = control-ref of="Current VI Reference"() -> (w140:refnum<vi>)
        n64 = Equal?(x=w139, y=T4."Closed" ("Front Panel Window:State")) -> (x = y?=w137:bool)
        n65 = Equal?(x=w145, y=T5."Run Time System" ("Application:Kind")) -> (x = y?=w143:bool)
        n66 = Or(x=w137, y=w143) -> (x .or. y?=w141:bool)
        n67 = Bundle By Name(cluster=w142, "Core.Current VI Reference"=w140, "Core.Close Panel on Exit?"=w141) -> (w147:T7)
        n68 = call <vilib>:"Add State(s) to Queue__jki_lib_state_machine.vi"("State(s) in (\"\")"=w149) -> ("States Out"=w148:string)  [unwired: 14 in]
      }
      frame "Error Handler" {
        # "Unhandled Error -- Display it"
        # "Handle any errors here.\nYou can also output any states to clean-up after errors occur"
        # "Clear error"
        n69 = call <vilib>:"General Error Handler.vi"("error in (no error)"=w151) -> ()  [unwired: 10 in, 5 out]
        n70 = call <vilib>:"Add State(s) to Queue__jki_lib_state_machine.vi"("State(s) in Front (\"\")"="/* Post Error States", "State(s) in (\"\")"=w155) -> ("States Out"=w154:string)  [unwired: 13 in]
      }
      frame "Exit" {
        # "Do not put any code in this frame.\n(No errors that occur here will be handled.)"
        n71 = call <vilib>:"Add State(s) to Queue__jki_lib_state_machine.vi"("State(s) in (\"\")"=w160) -> ("States Out"=w159:string)  [unwired: 14 in]
      }
      frame "---------- Data ----------" {
        # "Do not put any code in this frame.\n(It is a separator no-op. You can make a copy of this frame to create a new Data frame)"
        n72 = call <vilib>:"Add State(s) to Queue__jki_lib_state_machine.vi"("State(s) in (\"\")"=w164) -> ("States Out"=w163:string)  [unwired: 14 in]
      }
      frame "Data: Initialize" {
        w175 = string[][] []  # Temporary Preset
        w177 = T8 {"Current VI Reference"=refnum, "Close Panel on Exit?"=FALSE}  # Core
        w179 = TRUE  # Your Boolean data
        w178 = ""  # Your string data
        # "do not delete - used by framework"
        # "Add new data here."
        # "Data names and types of shift register data are defined by this bundle."
        # "Initialize the shift-register data, here.\n(data names are defined by what you wire into the bundle function)"
        n73 = local read "Preset Table Control"() -> (w174:string[][])
        n74 = property on="Headers" class="Tbl (strict)"() -> ("Column Headers[]"=w176:string[])  [unwired: 2 in, 2 out]
        n75 = local read "Queue Table Control"() -> (w173:string[][])
        n76 = call "PresetExecutionDataCluster.vi"() -> ("Preset Manager Cluster"=w172:T9)  [unwired: 1 in]
        n77 = Bundle("Core"=w177, "Your Boolean data"=w179, "Your string data"=w178, "Preset Table Control"=w174, "Column Headers[]"=w176, "Temporary Preset"=w175, "Queue Table Control"=w173, "Preset Manager Cluster"=w172) -> (w171:T7)  [unwired: 1 in]
        n78 = call <vilib>:"Add State(s) to Queue__jki_lib_state_machine.vi"("State(s) in (\"\")"=w182) -> ("States Out"=w181:string)  [unwired: 14 in]
        n79 = Bundle By Name(cluster=w171, "Preset Manager Cluster.DevStatusQueue"="DevStatusQueue", "Preset Manager Cluster.Experiment Name"="Experiment Name", "Preset Manager Cluster.Software Root"="Software Root", "Preset Manager Cluster.Filtered Devices List"="Filtered Devices List", "Preset Manager Cluster.Virtual Devices List"="Virtual Devices List") -> (w170:T7)
      }
      frame "Data: Cleanup" {
        # "Cleanup any data and references, here.\n(this is called automatically, by the Macro: Exit)"
        n80 = Unbundle By Name(w183) -> ("Core.Current VI Reference"=w186:refnum<vi>)
        n81 = Close Reference(reference=w186, error in (no error)=w185) -> (error out=w184:errorcluster)
        n82 = call <vilib>:"Add State(s) to Queue__jki_lib_state_machine.vi"("State(s) in (\"\")"=w188) -> ("States Out"=w187:string)  [unwired: 14 in]
      }
      frame "---------- UI ----------" {
        # "Do not put any code in this frame.\n(It is a separator no-op. You can make a copy of this frame to create a new UI frame)"
        n83 = call <vilib>:"Add State(s) to Queue__jki_lib_state_machine.vi"("State(s) in (\"\")"=w192) -> ("States Out"=w191:string)  [unwired: 14 in]
      }
      frame "UI: Initialize" {
        # "Initialize the User Interface, here.\n(this is called automatically, by the Macro: Init)"
        n84 = call <vilib>:"Add State(s) to Queue__jki_lib_state_machine.vi"("State(s) in (\"\")"=w196) -> ("States Out"=w195:string)  [unwired: 14 in]
      }
      frame "UI: Cursor Set" {
        # "Argument"
        # "Set and Unset Cursor Busy.\n(Usage: \"UI: Cursor Set >> Busy|Idle\")"
        n85 = case shown="\"Idle\", Default" w197 {
          tunnel: w199 -> [w204 w206]
          tunnel: [w203 w205] -> w198
          frame "Idle", Default {
            n86 = call <vilib>:"Unset Busy.vi"("error in (no error)"=w204) -> ("error out"=w203:errorcluster)  [unwired: 10 in]
          }
          frame "Busy" {
            n87 = call <vilib>:"Set Busy.vi"("error in (no error)"=w206) -> ("error out"=w205:errorcluster)  [unwired: 9 in, 1 out]
          }
        }
        n88 = call <vilib>:"Add State(s) to Queue__jki_lib_state_machine.vi"("State(s) in (\"\")"=w202) -> ("States Out"=w201:string)  [unwired: 14 in]
      }
      frame "UI: Front Panel State" {
        # "Argument"
        # "Set Front Panel Open or Closed\n(Usage: \"UI: Front Panel State >> Open|Close\")"
        n89 = Unbundle By Name(w209) -> ("Core.Current VI Reference"=w208:refnum<vi>)
        n90 = case shown="\"Minimize\", \"Minimized\"" w207 {
          tunnel: w211 -> [w219 w234 w245 w258 w271]
          tunnel: [w221 w235 w247 w260 w273] -> w210
          tunnel: w208 -> [w220 w232 w246 w259 w272]
          frame "Open", "Standard", Default {
            w214 = T4."Standard" ("State")
            n91 = property class="VI"(reference=w220, error in=w219) -> (reference out=w217:refnum<vi>, error out=w218:errorcluster, "FP.State"=w216:T4)
            n92 = Not Equal?(x=w216, y=w214) -> (x != y?=w215:bool)
            n93 = case shown="True" w215 {
              tunnel: [w225 w227] -> w221
              tunnel: w218 -> [w224 w227]
              tunnel: w217 -> [w223 _]
              tunnel: w214 -> [w222 _]
              frame True {
                n94 = invoke class="VI" method="FP.Open"(reference=w223, error in=w224, "Activate"=TRUE, "State"=w222) -> (error out=w225:errorcluster)  [unwired: 1 in, 4 out]
              }
              frame False {
              }
            }
          }
          frame "Close", "Closed" {
            n95 = property class="VI"(reference=w232, error in=w234) -> (reference out=w231:refnum<vi>, error out=w233:errorcluster, "FP.State"=w229:T4)
            n96 = Not Equal?(x=w229, y=T4."Closed" ("Front Panel Window:State")) -> (x != y?=w228:bool)
            n97 = case shown="True" w228 {
              tunnel: [w236 w239] -> w235
              tunnel: w233 -> [w236 w238]
              tunnel: w231 -> [_ w237]
              frame False {
              }
              frame True {
                n98 = invoke class="VI" method="FP.Close"(reference=w237, error in=w238) -> (error out=w239:errorcluster)  [unwired: 1 in, 2 out]
              }
            }
          }
          frame "Hidden", "Hide" {
            w240 = T4."Hidden" ("State")
            n99 = property class="VI"(reference=w246, error in=w245) -> (reference out=w243:refnum<vi>, error out=w244:errorcluster, "FP.State"=w242:T4)
            n100 = Not Equal?(x=w242, y=w240) -> (x != y?=w241:bool)
            n101 = case shown="True" w241 {
              tunnel: [w251 w252] -> w247
              tunnel: w244 -> [w250 w252]
              tunnel: w243 -> [w249 _]
              tunnel: w240 -> [w248 _]
              frame True {
                n102 = invoke class="VI" method="FP.Open"(reference=w249, error in=w250, "State"=w248) -> (error out=w251:errorcluster)  [unwired: 2 in, 4 out]
              }
              frame False {
              }
            }
          }
          frame "Minimize", "Minimized" {
            w253 = T4."Minimized" ("State")
            n103 = property class="VI"(reference=w259, error in=w258) -> (reference out=w256:refnum<vi>, error out=w257:errorcluster, "FP.State"=w255:T4)
            n104 = Not Equal?(x=w255, y=w253) -> (x != y?=w254:bool)
            n105 = case shown="True" w254 {
              tunnel: [w264 w265] -> w260
              tunnel: w257 -> [w263 w265]
              tunnel: w256 -> [w262 _]
              tunnel: w253 -> [w261 _]
              frame True {
                n106 = invoke class="VI" method="FP.Open"(reference=w262, error in=w263, "State"=w261) -> (error out=w264:errorcluster)  [unwired: 2 in, 4 out]
              }
              frame False {
              }
            }
          }
          frame "Maximize", "Maximized" {
            w266 = T4."Maximized" ("State")
            n107 = property class="VI"(reference=w272, error in=w271) -> (reference out=w269:refnum<vi>, error out=w270:errorcluster, "FP.State"=w268:T4)
            n108 = Not Equal?(x=w268, y=w266) -> (x != y?=w267:bool)
            n109 = case shown="True" w267 {
              tunnel: [w277 w278] -> w273
              tunnel: w270 -> [w276 w278]
              tunnel: w269 -> [w275 _]
              tunnel: w266 -> [w274 _]
              frame True {
                n110 = invoke class="VI" method="FP.Open"(reference=w275, error in=w276, "State"=w274) -> (error out=w277:errorcluster)  [unwired: 2 in, 4 out]
              }
              frame False {
              }
            }
          }
        }
        n111 = call <vilib>:"Add State(s) to Queue__jki_lib_state_machine.vi"("State(s) in (\"\")"=w213) -> ("States Out"=w212:string)  [unwired: 14 in]
      }
      frame "---------- Macro ----------" {
        # "Do not put any code in this frame.\n(It is a separator no-op. You can make a copy of this frame to create a new Macro frame)"
        n112 = call <vilib>:"Add State(s) to Queue__jki_lib_state_machine.vi"("State(s) in (\"\")"=w282) -> ("States Out"=w281:string)  [unwired: 14 in]
      }
      frame "Macro: Initialize" {
        w283 = "Data: Initialize\nInitialize Core Data\nUI: Initialize\nUI: Front Panel State >> Open\nInitialize UDP Variables"  # Data: Initialize Initialize Core Data UI: Initialize UI: Front Panel State >> Open Initialize UDP Variables
        # "Initialization Macro\n(This is called once, when the VI starts)"
        n113 = call <vilib>:"Add State(s) to Queue__jki_lib_state_machine.vi"("State(s) in Front (\"\")"=w283, "State(s) in (\"\")"=w287) -> ("States Out"=w286:string)  [unwired: 13 in]
      }
      frame "Macro: Exit" {
        # "Exit Macro\n(This is called once, when the VI exits)"
        n114 = Unbundle By Name(w294) -> ("Core.Close Panel on Exit?"=w293:bool)
        n115 = Select(t="UI: Front Panel State >> Close", s=w293, f="") -> (s? t:f=w290:string)
        n116 = call <vilib>:"Add State(s) to Queue__jki_lib_state_machine.vi"("State(s) in (\"\")"=w290, "State(s) at Back (\"\")"="Data: Cleanup\nExit") -> ("States Out"=w288:string)  [unwired: 13 in]
        n117 = call <vilib>:"Add State(s) to Queue__jki_lib_state_machine.vi"("State(s) in Front (\"\")"=w288, "State(s) in (\"\")"=w297) -> ("States Out"=w296:string)  [unwired: 13 in]
      }
      frame "Initialize UDP Variables" {
        # "Do not put any code in this frame.\n(It is a separator no-op. You can make a copy of this frame to create a new Macro frame)"
        n118 = Unbundle By Name(w306) -> ("Preset Manager Cluster.Experiment Name"=w304:string)
        n119 = call "UPD Variable Init.vi"("Expt Name"=w304) -> ("Mcast Address"=w300:string, "UDP timeout ms"=w301:i32, "MC Multicast"=w302:refnum<k16>, "My IP"=w303:string, "Mcast remote"=w299:u16, "> Name, devtype, ip, dev comm port, class, location for all devices>"=w298:string[][])  [unwired: 5 in]
        n120 = call <vilib>:"Add State(s) to Queue__jki_lib_state_machine.vi"("State(s) in (\"\")"=w309) -> ("States Out"=w308:string)  [unwired: 14 in]
        n121 = Bundle By Name(cluster=w306, "Preset Manager Cluster.My IP"=w303, "Preset Manager Cluster.MC Multicast"=w302, "Preset Manager Cluster.UDP timeout ms"=w301, "Preset Manager Cluster.Mcast address"=w300, "Preset Manager Cluster.MCast Remote"=w299, "Preset Manager Cluster.All Devices Core Info"=w298) -> (w305:T7)
      }
      frame "---------- New Category ----------" {
        # "Template Separator\n(You can make a copy of, or modify, this frame)"
        n122 = call <vilib>:"Add State(s) to Queue__jki_lib_state_machine.vi"("State(s) in (\"\")"=w313) -> ("States Out"=w312:string)  [unwired: 14 in]
      }
      frame "Compare Table" {
        # "Template Separator\n(You can make a copy of, or modify, this frame)"
        n123 = property on="PRESET FROM DB" class="Tbl (strict)"() -> ("Value"=w320:string[][])  [unwired: 2 in, 2 out]
        n124 = property on="ECS File" class="Tbl (strict)"() -> ("Value"=w319:string[][])  [unwired: 2 in, 2 out]
        n125 = call "Left Join.vi"("Array 2"=w319, "Array 1"=w320) -> ("Left Joined Array"=w317:string[][])  [unwired: 9 in]
        n126 = call <vilib>:"Add State(s) to Queue__jki_lib_state_machine.vi"("State(s) in Front (\"\")"="Table Update" ("State(s) in Front (\"\")"), "State(s) in (\"\")"=w323) -> ("States Out"=w322:string)  [unwired: 13 in]
        n127 = Bundle By Name(cluster=w318, "Preset Table Control"=w317, "Column Headers[]"=string[] ["Device Name", "Device Variable", "Preset Value", "ECS Value"] ("Column Headers")) -> (w316:T7)
      }
      frame "Choose Values" {
        # "Template Separator\n(You can make a copy of, or modify, this frame)"
        n128 = property on="Preset Table Control" class="Tbl (strict)"() -> ("Value"=w327:string[][])  [unwired: 2 in, 2 out]
        n129 = call "Value_Selection_in_Table_GUI.vi"("Column Headers"=string[] ["Device Name", "Device Variable", "Preset Value", "ECS Value"], "SELECTION TABLE - Click on values to keep"=w327) -> ("Coordinate Array"=→"Coordinate Array":i32[][])  [unwired: 9 in]
        n130 = call <vilib>:"Add State(s) to Queue__jki_lib_state_machine.vi"("State(s) in Front (\"\")"="Implement Value Change" ("State(s) in Front (\"\")"), "State(s) in (\"\")"=w331) -> ("States Out"=w330:string)  [unwired: 13 in]
      }
      frame "Implement Value Change" {
        # "Template Separator\n(You can make a copy of, or modify, this frame)"
        n131 = Unbundle By Name(w337) -> ("Preset Table Control"=w335:string[][])
        n132 = property on="Coordinate Array" class="Arr (strict)"() -> ("Value"=w334:i32[][])  [unwired: 2 in, 2 out]
        n133 = call "Value_Update_to_Preset.vi"("Coordinate Array with Changes"=w334, "Input Table"=w335) -> ("Column Headers"=w332:string[], "Output Table with Changes"=w333:string[][])  [unwired: 8 in]
        n134 = Bundle By Name(cluster=w337, "Preset Table Control"=w333, "Column Headers[]"=w332) -> (w336:T7)
        n135 = call <vilib>:"Add State(s) to Queue__jki_lib_state_machine.vi"("State(s) in Front (\"\")"="Table Update" ("State(s) in Front (\"\")"), "State(s) in (\"\")"=w341) -> ("States Out"=w340:string)  [unwired: 13 in]
      }
      frame "Load Preset from DB" {
        # "Template Separator\n(You can make a copy of, or modify, this frame)"
        n136 = property on="Preset Menu" class="Ring (strict)"() -> ("RingText.Text"=w344:string)  [unwired: 2 in, 2 out]
        n137 = call "Preset_to_Array.vi"("Preset Name"=w344) -> ("Column Headers"=w343:string[], "Preset Table"=w342:string[][])  [unwired: 9 in]
        "PRESET FROM DB" <- w342
        n138 = Bundle By Name(cluster=w347, "Preset Table Control"=w342, "Column Headers[]"=w343) -> (w346:T7)
        n139 = call <vilib>:"Add State(s) to Queue__jki_lib_state_machine.vi"("State(s) in Front (\"\")"="Table Update" ("State(s) in Front (\"\")"), "State(s) in (\"\")"=w350) -> ("States Out"=w349:string)  [unwired: 13 in]
      }
      frame "Load Configuration File" {
        # "Template Separator\n(You can make a copy of, or modify, this frame)"
        n140 = call "Configuration_to_Array.vi"("file (use dialog)"="Navigate to ECS File") -> ("Table Control"=w353:string[][])  [unwired: 10 in]
        "ECS File" <- w353
        n141 = Bundle By Name(cluster=w355, "Preset Table Control"=w353, "Column Headers[]"=string[] ["Device Name", "Device Variable", "ECS Values"] ("Column Headers")) -> (w354:T7)
        n142 = call <vilib>:"Add State(s) to Queue__jki_lib_state_machine.vi"("State(s) in Front (\"\")"="Table Update" ("State(s) in Front (\"\")"), "State(s) in (\"\")"=w359) -> ("States Out"=w358:string)  [unwired: 13 in]
      }
      frame "Save Preset" {
        # "Template Separator\n(You can make a copy of, or modify, this frame)"
        n143 = call <vilib>:"Three Button Dialog.vi"("Right Button Text (\"Cancel\")"="Cancel" ("Right Button Text (\"Cancel\")"), "Center Button Text (\"No\")"="Overwrite Existing Preset" ("Right Button Text (\"Cancel\")"), "Left Button Text (\"Yes\")"="Save as New Preset" ("Left Button Text (\"Yes\")"), "message"="Save the current preset as - ") -> ("Which Button?"=w361:T10)  [unwired: 7 in]
        n144 = case shown="\"Right Button\", Default" w361 {
          tunnel: ["Save as New Preset" ("State(s) in Front (\"\")") "Overwrite Existing Preset" ("Right Button Text (\"Cancel\")") _] -> w360
          frame "Left Button" {
          }
          frame "Center Button" {
          }
          frame "Right Button", Default {
          }
        }
        n145 = call <vilib>:"Add State(s) to Queue__jki_lib_state_machine.vi"("State(s) in Front (\"\")"=w360, "State(s) in (\"\")"=w369) -> ("States Out"=w368:string)  [unwired: 13 in]
      }
      frame "Save as New Preset" {
        # "Template Separator\n(You can make a copy of, or modify, this frame)"
        n146 = call "Preset Name"() -> ("Name"=w373:string, "OK"=w382:bool)  [unwired: 17 in, 1 out]
        n147 = property on="Preset Menu" class="Ring (strict)"() -> ("Strings []"=w379:string[])  [unwired: 2 in, 2 out]
        n148 = Search 1D Array(1D array=w379, element=w373) -> (index of element=w378:i32)  [unwired: 1 in]
        n149 = call <vilib>:"Trim Whitespace.vi"("string"=w373) -> ("trimmed string"=w381:string)  [unwired: 1 in]
        n150 = Equal?(x=w381, y="") -> (x = y?=w376:bool)
        n151 = Not Equal?(x=w378, y=-1) -> (x != y?=w375:bool)
        n152 = Or(x=w376, y=w375) -> (x .or. y?=w374:bool)
        n153 = case shown="True" w382 {
          tunnel: w374 -> [_ w388]
          tunnel: w373 -> [_ w387]
          frame False {
          }
          frame True {
            n154 = case shown="False" w388 {
              tunnel: w387 -> [w389 _]
              frame False {
                n155 = stacked-sequence {
                  tunnel: w389 -> [w391]
                  frame #0 {
                    n156 = local read "Preset Table Control"() -> (w390:string[][])
                    n157 = for {
                      tunnel: w391 -> [w396]
                      tunnel: w390 -> [w392] mode=indexing
                      n158 = Insert Into Array(array=w392, index=0, new element=w396) -> (w394:string[])
                      n159 = call "SQL Insert null.vi"("Values"=w394, "Column Names"=string[] ["presetName", "presetDevice", "presetVariable", "presetValue"], "Table"="Presets") -> ("Query String"=w393:string)  [unwired: 8 in]
                      n160 = disable-structure shown="Enabled" {
                        disable-tunnel: w393 -> [w399 _]
                        frame Enabled {
                          n161 = call "SQL Server Info.vi"() -> ("SQL Server Info"=w400:T12)
                          n162 = call "SQL Query.vi"("SQL Server Info"=w400, "Query"=w399) -> ()  [unwired: 8 in, 2 out]
                        }
                        frame Disabled {
                        }
                      }
                    }
                  }
                }
              }
              frame True {
                n163 = One Button Dialog(message="Name field was blank or the Preset Name already exists") -> ()  [unwired: 1 in, 1 out]
              }
            }
          }
        }
        n164 = call <vilib>:"Add State(s) to Queue__jki_lib_state_machine.vi"("State(s) in Front (\"\")"="Load Preset from DB>>Table Update" ("State(s) in Front (\"\")"), "State(s) in (\"\")"=w386) -> ("States Out"=w385:string)  [unwired: 13 in]
      }
      frame "Overwrite Existing Preset" {
        # "Template Separator\n(You can make a copy of, or modify, this frame)"
        n165 = property on="Preset Menu" class="Ring (strict)"() -> ("RingText.Text"=w403:string)  [unwired: 2 in, 2 out]
        n166 = Concatenate Strings("Are you sure you want to overwrite " ("string"), w403, " with the current table ?" ("string")) -> (w406:string)
        n167 = Two Button Dialog(message=w406, 2:"Yes" ("T button name (\"OK\")")) -> (T button?=w404:bool)  [unwired: 1 in]
        n168 = case shown="True" w404 {
          tunnel: w403 -> [_ w413]
          frame False {
          }
          frame True {
            n169 = stacked-sequence {
              seq-local: [w414 _] -> [_ w424]
              tunnel: w413 -> [w415 w423]
              tunnel: [_ w424] -> _
              frame #0 {
                n170 = disable-structure shown="Enabled" {
                  disable-tunnel: w415 -> [w419 _]
                  disable-tunnel: [w416 _] -> w414
                  frame Enabled {
                    n171 = Concatenate Strings("DELETE FROM Presets WHERE presetName='", w419, "'" ("string")) -> (w417:string)
                    n172 = call "SQL Server Info.vi"() -> ("SQL Server Info"=w421:T12)
                    n173 = call "SQL Query.vi"("SQL Server Info"=w421, "Query"=w417) -> ("error out"=w416:errorcluster)  [unwired: 8 in, 1 out]
                  }
                  frame Disabled {
                  }
                }
              }
              frame #1 {
                n174 = local read "Preset Table Control"() -> (w422:string[][])
                n175 = for {
                  tunnel: w424 -> [w432]
                  tunnel: w423 -> [w429]
                  tunnel: w422 -> [w425] mode=indexing
                  n176 = Insert Into Array(array=w425, index=0, new element=w429) -> (w427:string[])
                  n177 = call "SQL Insert null.vi"("Values"=w427, "Column Names"=string[] ["presetName", "presetDevice", "presetVariable", "presetValue"], "Table"="Presets") -> ("Query String"=w426:string)  [unwired: 8 in]
                  n178 = disable-structure shown="Enabled" {
                    disable-tunnel: w432 -> [w434 _]
                    disable-tunnel: w426 -> [w433 _]
                    frame Enabled {
                      n179 = call "SQL Server Info.vi"() -> ("SQL Server Info"=w435:T12)
                      n180 = call "SQL Query.vi"("error in (no error)"=w434, "SQL Server Info"=w435, "Query"=w433) -> ()  [unwired: 7 in, 2 out]
                    }
                    frame Disabled {
                    }
                  }
                }
              }
            }
          }
        }
        n181 = call <vilib>:"Add State(s) to Queue__jki_lib_state_machine.vi"("State(s) in Front (\"\")"="Load Preset from DB>>Table Update" ("State(s) in Front (\"\")"), "State(s) in (\"\")"=w412) -> ("States Out"=w411:string)  [unwired: 13 in]
      }
      frame "Delete Preset" {
        # "Template Separator\n(You can make a copy of, or modify, this frame)"
        n182 = property on="Preset Menu" class="Ring (strict)"() -> ("RingText.Text"=w436:string)  [unwired: 2 in, 2 out]
        n183 = Concatenate Strings("Are you sure you want to delete " ("string"), w436, ". NOTE - THIS ACTION IS NOT REVERSIBLE" ("string")) -> (w439:string)
        n184 = Two Button Dialog(message=w439, 2:"Yes" ("T button name (\"OK\")")) -> (T button?=w437:bool)  [unwired: 1 in]
        n185 = case shown="True" w437 {
          tunnel: w436 -> [_ w447]
          frame False {
          }
          frame True {
            n186 = stacked-sequence {
              tunnel: w447 -> [w448]
              frame #0 {
                n187 = disable-structure shown="Disabled" {
                  disable-tunnel: w448 -> [w453 _]
                  frame Disabled {
                    n188 = Concatenate Strings("DELETE FROM Presets WHERE presetName='", w453, "'" ("string")) -> (w449:string)
                    n189 = call "SQL Server Info.vi"() -> ("SQL Server Info"=w452:T12)
                    n190 = call "SQL Query.vi"("SQL Server Info"=w452, "Query"=w449) -> ()  [unwired: 8 in, 2 out]
                  }
                  frame Enabled {
                  }
                }
              }
            }
          }
        }
        n191 = call <vilib>:"Add State(s) to Queue__jki_lib_state_machine.vi"("State(s) in Front (\"\")"="Load Preset from DB>>Table Update" ("State(s) in Front (\"\")"), "State(s) in (\"\")"=w446) -> ("States Out"=w445:string)  [unwired: 13 in]
      }
      frame "Execute Preset" {
        # "Template Separator\n(You can make a copy of, or modify, this frame)"
        n192 = call <vilib>:"Add State(s) to Queue__jki_lib_state_machine.vi"("State(s) in Front (\"\")"="Load Preset from DB\nTable Update\nMC Control Update\nSend preset Command" ("State(s) in Front (\"\")"), "State(s) in (\"\")"=w458) -> ("States Out"=w457:string)  [unwired: 13 in]
      }
      frame "New Category: 1" {
        # "Your code here.\n(You can make a copy of, or modify, this frame)"
        n193 = call <vilib>:"Add State(s) to Queue__jki_lib_state_machine.vi"("State(s) in (\"\")"=w462) -> ("States Out"=w461:string)  [unwired: 14 in]
      }
      frame "New Category: 2" {
        # "Your code here.\n(You can make a copy of, or modify, this frame)"
        n194 = call <vilib>:"Add State(s) to Queue__jki_lib_state_machine.vi"("State(s) in (\"\")"=w466) -> ("States Out"=w465:string)  [unwired: 14 in]
      }
      frame "-------Table Update--------" {
        # "Template Separator\n(You can make a copy of, or modify, this frame)"
        n195 = call <vilib>:"Add State(s) to Queue__jki_lib_state_machine.vi"("State(s) in (\"\")"=w470) -> ("States Out"=w469:string)  [unwired: 14 in]
      }
      frame "Table Update" {
        # "Template Separator\n(You can make a copy of, or modify, this frame)"
        n196 = Unbundle By Name(w473) -> ("Preset Table Control"=w472:string[][], "Column Headers[]"=w471:string[])
        n197 = call <vilib>:"Add State(s) to Queue__jki_lib_state_machine.vi"("State(s) in (\"\")"=w476) -> ("States Out"=w475:string)  [unwired: 14 in]
        n198 = property on="Preset Table Control" class="Tbl (strict)"("Value"=w472, "Column Headers[]"=w471) -> ()  [unwired: 2 in, 2 out]
      }
      frame "--------Queue Presets------------" {
        # "Template Separator\n(You can make a copy of, or modify, this frame)"
        n199 = call <vilib>:"Add State(s) to Queue__jki_lib_state_machine.vi"("State(s) in (\"\")"=w480) -> ("States Out"=w479:string)  [unwired: 14 in]
      }
      frame "Init: Queue Preset" {
        # "Template Separator\n(You can make a copy of, or modify, this frame)"
        n200 = property on="Tab Control" class="TabCtl (strict)"() -> ("Value"=w481:T1)  [unwired: 2 in, 2 out]
        n201 = Equal?(x=w481, y=1) -> (x = y?=w484:bool)
        n202 = case shown="False" w484 {
          frame False {
          }
          frame True {
            n203 = call "preset SQL Queries.vi"("Preset Query"=Preset_Query_Enum."GetAllPresetNames") -> ("data"=w488:string[][])  [unwired: 8 in, 2 out]
            n204 = Array Subset(array=w488, index (row)=1 ("index")) -> (w489:string[][])  [unwired: 3 in]
            n205 = property on="Queue Table Control" class="Tbl (strict)"("Value"=w489) -> ()  [unwired: 2 in, 2 out]
          }
        }
        n206 = call <vilib>:"Add State(s) to Queue__jki_lib_state_machine.vi"("State(s) in (\"\")"=w487) -> ("States Out"=w486:string)  [unwired: 14 in]
      }
      frame "Reset Queue" {
        # "Template Separator\n(You can make a copy of, or modify, this frame)"
        n207 = property on="Queue Table" class="Tbl (strict)"("Value"=string[][] [] ("Queue Table")) -> ()  [unwired: 2 in, 2 out]
        n208 = call <vilib>:"Add State(s) to Queue__jki_lib_state_machine.vi"("State(s) in (\"\")"=w496) -> ("States Out"=w495:string)  [unwired: 14 in]
      }
      frame "Execute Queue" {
        # "Template Separator\n(You can make a copy of, or modify, this frame)"
        n209 = property on="Queue Table" class="Tbl (strict)"() -> ("Value"=w500:string[][])  [unwired: 2 in, 2 out]
        n210 = Index Array(array=w500, index (col)=0 ("disabled index (col)")) -> (element=w497:string[])  [unwired: 1 in]
        n211 = Array Size(array=w497) -> (size(s)=w498:i32)
        n212 = for {
          N: w498 -> [_]
          tunnel: w497 -> [w506] mode=indexing
          i -> [w507]
          n213 = flat-sequence {
            tunnel: [w510] -> w509
            tunnel: w507 -> [w511]
            tunnel: w506 -> [w510]
            tunnel: [w516] -> w508
            tunnel: w509 -> [w516]
            tunnel: w508 -> [w518]
            frame #0 {
              n214 = property on="Queue Table" class="Tbl (strict)"() -> ("Value"=w512:string[][])  [unwired: 2 in, 2 out]
              n215 = Index Array(array=w512, index (row)=w511, index (col)=0 ("disabled index (col)")) -> ()  [unwired: 1 out]
              n216 = local read "Outgoing Preset Refnum"() -> (w514:refnum<vi>)
              n217 = property class="Str"(reference=w514, "Val(Sgnl)"=w510) -> ()  [unwired: 1 in, 2 out]
            }
            frame #1 {
              n218 = local read "Execute Preset Refnum"() -> (w515:refnum<vi>)
              n219 = property class="Ctl"(reference=w515, "Val(Sgnl)"=TRUE) -> ()  [unwired: 1 in, 2 out]
            }
            frame #2 {
              n220 = while {
                tunnel: w518 -> [w522]
                stop <- w521 stop-if-true
                n221 = local read "Incoming Preset Refnum"() -> (w519:refnum<vi>)
                n222 = property class="Str"(reference=w519) -> ("Value"=w523:string)  [unwired: 1 in, 2 out]
                n223 = Equal?(x=w523, y=w522) -> (x = y?=w521:bool)
                n224 = Wait (ms)(milliseconds to wait=u32 10) -> ()  [unwired: 1 out]
              }
            }
          }
        }
        n225 = call <vilib>:"Add State(s) to Queue__jki_lib_state_machine.vi"("State(s) in Front (\"\")"="Table Update" ("State(s) in Front (\"\")"), "State(s) in (\"\")"=w505) -> ("States Out"=w504:string)  [unwired: 13 in]
      }
      frame "-------Preset Execution----------" {
        # "Template Separator\n(You can make a copy of, or modify, this frame)"
        n226 = call <vilib>:"Add State(s) to Queue__jki_lib_state_machine.vi"("State(s) in (\"\")"=w527) -> ("States Out"=w526:string)  [unwired: 14 in]
      }
      frame "MC Control Update" {
        # "Template Separator\n(You can make a copy of, or modify, this frame)"
        n227 = Bundle By Name(cluster=w535, "Preset Manager Cluster.My IP"="My IP", "Preset Manager Cluster.Mcast address"="Mcast address", "Preset Manager Cluster.MCast Remote"="MCast Remote", "Preset Manager Cluster.UDP timeout ms"="UDP timeout ms", "Preset Manager Cluster.MC Multicast"="MC Multicast", "Preset Manager Cluster.All Devices Core Info"="All Devices Core Info") -> (w528:T7)
        n228 = call <vilib>:"Add State(s) to Queue__jki_lib_state_machine.vi"("State(s) in (\"\")"=w538) -> ("States Out"=w537:string)  [unwired: 14 in]
      }
      frame "General wait" {
        # "Template Separator\n(You can make a copy of, or modify, this frame)"
        n229 = call "get arguments of jki state.vi"("jki arguments"=w539) -> ("Arg 1"=w541:string)  [unwired: 1 in, 2 out]
        n230 = Decimal String To Number(string=w541) -> (number=w540:i32)  [unwired: 2 in, 1 out]
        n231 = Wait (ms)(milliseconds to wait=w540) -> ()  [unwired: 1 out]
        n232 = call <vilib>:"Add State(s) to Queue__jki_lib_state_machine.vi"("State(s) in (\"\")"=w545) -> ("States Out"=w544:string)  [unwired: 14 in]
      }
      frame "Poll Devices" {
        # "rem virt devs"
        # "Template Separator\n(You can make a copy of, or modify, this frame)"
        n233 = Unbundle By Name(w559) -> ("Preset Manager Cluster"=w558:T9)
        n234 = Unbundle By Name(w558) -> ("PresetName"=w554:string, "Current Preset Devices"=w553:string[], "All Devices Core Info"=w557:string[][], "Filtered Devices List"=w556:string[], "Virtual Devices List"=w555:string[], "DevStatusQueue"=w548:refnum<queue>)
        n235 = call "search string array for elements in 2nd string array.vi"("search for"=w555, "search in"=w556) -> ("Indices of Elements"=w560:i32[])  [unwired: 9 in]
        n236 = call-poly <userlib>:"Delete Elements from Array__ogtk.vi"("indices"=w560, "array"=w556) -> ("array w/ subset deleted"=w550:string[])  [unwired: 8 in, 1 out]
        n237 = Preview Queue Element(queue=w548, timeout in ms (-1)=200) -> (element=w547:string[][], error out=→"error out":errorcluster)  [unwired: 1 in, 2 out]
        n238 = call "get info from core device data.vi"("devices to get data from"=w550, "All Devices Core Info"=w557) -> ("IP Addresses"=w551:string[])  [unwired: 2 in, 1 out]
        n239 = Empty Array?(array=w551) -> (empty?=w552:bool)
        n240 = case shown="False" w552 {
          tunnel: w554 -> [w569 _]
          tunnel: w553 -> [w568 _]
          tunnel: w551 -> [w567 _]
          tunnel: w550 -> [w566 _]
          tunnel: w547 -> [w564 _]
          frame False {
            (unwired) 200 ("timeout in ms (-1)")
            # "Determine which devices are ON/OFF"
            n241 = call "get device status from tcp data array.vi"("TCP Device status data"=w564, "Current Preset Devices"=w568, "IP Addresses in"=w567, "Filtered Device List"=w566, "Requested Preset"=w569) -> ("Device Errors"=→"Device Errors":string[][], "Active boolean array"=→"Active Device array":bool[], "preset diagnostics"=w570:T13, "Active IP Addresses"=→"Active Dev/IP":string[], "Devices Not alive"=→"Devices not started":string[])  [unwired: 3 in, 3 out]
            n242 = Unbundle By Name(w570) -> ("Active Preset Achieved"=w571:bool)
            n243 = Select(t=w569, s=w571, f="Undefined") -> (s? t:f=→"Active Preset":string)
          }
          frame True {
          }
        }
        n244 = call <vilib>:"Add State(s) to Queue__jki_lib_state_machine.vi"("State(s) in (\"\")"=w563) -> ("States Out"=w562:string)  [unwired: 14 in]
      }
      frame "Send Preset Command" {
        # "This State builds the Multicast Preset Command to all Devices"
        # "Template Separator\n(You can make a copy of, or modify, this frame)"
        n245 = property on="Preset Menu" class="Ring (strict)"() -> ("RingText.Text"=w583:string)  [unwired: 2 in, 2 out]
        n246 = Unbundle By Name(w581) -> ("Preset Manager Cluster.My IP"=w580:string)
        n247 = call "preset SQL Queries.vi"("Expt name / MCIP/ Variable/Preset Name"=w583, "Preset Query"=Preset_Query_Enum."GetPresetDeviceNames") -> ("1st column 1st data"=w578:string[])  [unwired: 7 in, 2 out]
        n248 = Concatenate Strings("preset>>" ("string"), w583, ">>" ("string"), w580) -> (w579:string)
        n249 = Bundle By Name(cluster=w581, "Preset Manager Cluster.PresetName"=w583, "Preset Manager Cluster.Mcast command"=w579, "Preset Manager Cluster.Current Preset Devices"=w578) -> (w582:T7)
        n250 = call <vilib>:"Add State(s) to Queue__jki_lib_state_machine.vi"("State(s) in (\"\")"=w589, "State(s) at Back (\"\")"="Send Multicast>>Empty\nGeneral wait>>10\nSend Multicast>>Empty\nGeneral wait>>40\nSend Multicast\nPoll Devices" ("Remaining States")) -> ("States Out"=w588:string)  [unwired: 13 in]
      }
      frame "Send Multicast" {
        # "Template Separator\n(You can make a copy of, or modify, this frame)"
        n251 = Unbundle By Name(w592) -> ("Preset Manager Cluster.MCast Remote"=w598:u16, "Preset Manager Cluster.Mcast address"=w597:string, "Preset Manager Cluster.UDP timeout ms"=w595:i32, "Preset Manager Cluster.Mcast command"=w594:string, "Preset Manager Cluster.MC Multicast"=w593:refnum<k16>)
        n252 = String To IP(1:w597) -> (0:w596:u32)
        n253 = UDP Write(address=w596, port or service name=w598, connection ID=w593, data in=w594, 9:w595) -> (3:w591:refnum<k16>)  [unwired: 1 in, 1 out]
        n254 = Bundle By Name(cluster=w592, "Preset Manager Cluster.MC Multicast"=w591) -> (w590:T7)
        n255 = call <vilib>:"Add State(s) to Queue__jki_lib_state_machine.vi"("State(s) in (\"\")"=w601) -> ("States Out"=w600:string)  [unwired: 14 in]
      }
    }
  }
